vi "Auto_calibrate.vi"(3 "Mode":T4, 5 "Traverse line":T5 {"Carrier_2 Q (l/min)" format="%#.2f"; "Row Duration (mins)" format="%#.1f"; "Row No" min=0; "Trace Gas Concentration (%)" min=0.0 format="%#_4f"; "Carrier_1 Q (l/min)" format="%#.2f"; "Tunnel Speed" format="%#.2f"; "Start X" format="%#.2f"; "Start Y" format="%#.2f"; "Start Z" format="%#.2f"; "End X" format="%#.2f"; "End Y" format="%#.2f"; "End Z" format="%#.2f"; "Averaging time (min)" min=0.0 format="%#.2f"}) -> (0 "Error Messages":string, 1 "Status":T2, 2 "Traverse Out":T5 {"Carrier_2 Q (l/min)" format="%#.2f"; "Row Duration (mins)" format="%#.1f"; "Row No" min=0; "Trace Gas Concentration (%)" min=0.0 format="%#_4f"; "Carrier_1 Q (l/min)" format="%#.2f"; "Tunnel Speed" format="%#.2f"; "Start X" format="%#.2f"; "Start Y" format="%#.2f"; "Start Z" format="%#.2f"; "End X" format="%#.2f"; "End Y" format="%#.2f"; "End Z" format="%#.2f"; "Averaging time (min)" min=0.0 format="%#.2f"})   [LabVIEW 2015]
uses:
  Gen Trav/Traverse_cluster.ctl
  Gen Trav/Spacing.ctl
  Controls/Multi_run_mode.ctl
  Controls/User_Specific_mode.ctl
  Controls/Auto_Calib_Type.ctl
  Gen Trav/Multi_Run_Status.ctl
  Controls/Auto_Calib_Case.ctl
  File/Setup_Filetype.ctl
  Calibration/Calib_mode.ctl
  ADAM Client/Sub VIs/ADAM Controls/Valco_valve_ph.ctl
  ADAM Client/Sub VIs/ADAM Controls/Client_Source_Status.ctl
  Controls/Setup.ctl
  Controls/Post_Process.ctl
  Controls/Save_Data.ctl
  Controls/App_Global.ctl
  <vilib>/Analysis/baseanly.llb/Mean (DBL).vi
  Globals/Preference_global.vi
  Globals/Meas_global.vi
  Globals/Calib_global.vi
  Globals/Trav_pos_global.vi
  Globals/Gas_management_global.vi
  Globals/Extra_Commands_Global.vi
  <vilib>/Analysis/NI_AALBase.lvlib
  <vilib>/Analysis/NI_AALPro.lvlib
panel:
  out "Mix_own_Calib_Gases":bool
  out "Slope":dbl[](array[numeric])
  out "Minimum St Dev":dbl[](array[numeric])
  out "Wait factor":dbl
  out "Orig Calib file string":string
  out "Concentrations":dbl[](array[numeric])
  out "FFID St Dev":dbl[][](array[numeric]) format="%.2f"
  in  "Clear Calib History":bool
  out "Coefficients":dbl[][](array[numeric]) format="%.2f"
  out "Currently in Case":T1
  out "Valve position":dbl format="%.2f"
  out "Currently On":i32
  out "Values":dbl[][](array[numeric]) format="%.2f"
  out "FF Indexes":i16[](array[numeric])
  out "Ch No's":i16[](array[numeric])
  out "No of Calib Points":i32
  out "Root Name":string[](array[string])
  out "Calibration varying":T3
  in  "stop":bool
  out "New Calib Filenames":path[](array[path])
  # "Specific Argument Options\n      Tunnel Speed;1;2;3;4\nOR  Traverse Position\nOR   Concentration"
  # "X           Y            Z"
  # "Start"
  # "End"
  # "X           Y            Z"
  # "Start"
  # "End"
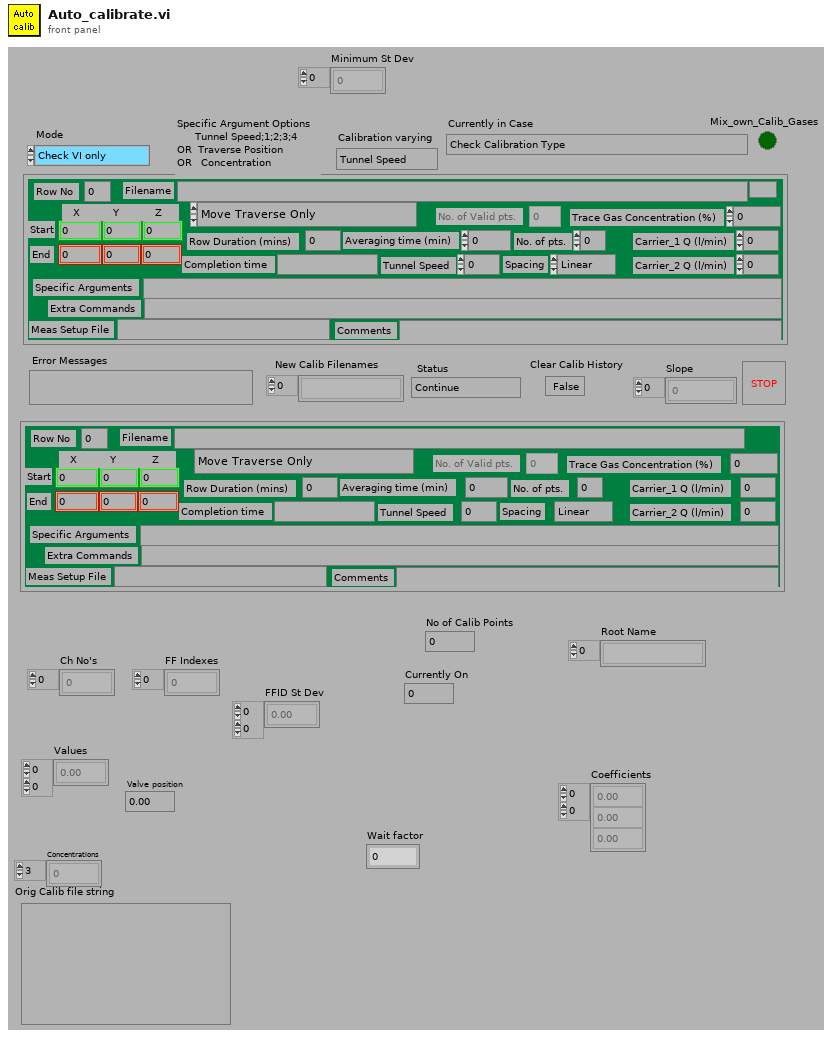
[diagram p1: front panel]
types:
  T1 = typedef "Auto_Calib_Case.ctl" = enum16{"Check Calibration Type", "Check if Original Calib file is Valid", "Get sampling rate etc. from meas setup file", "Setup Calibration Program", "Get Channel Numbers", "Check use latest selected on Mesurement setup files", "Create New Calib Filenames", "Setup Calibration Values in 2D array", "Create Measurement Setup File (Concentration Only)", "Are There Enough Calibration Points", "Set Measurement Conditions", "Measure Calibration Point", "Do Another Calibration Point?", "Skip Next Frame?", "Insert New calibration Filenames into Measurement Setup file", "Warn if FFID calibration is very non linear", "Warn if FFID variance is high", "Insert Bkgnd Variance into calib file", "Warn if FFID voltages are too low", "Warn if Current Calibration fit is poor", "Warn if Calibration Coefficients have significantly altered", "End"}
  T2 = typedef "Multi_Run_Status.ctl" = enum16{"Continue", "Jump to Next Point", "Jump to Next Row", "Jump To Fall Back", "Terminate Run"}
  T3 = typedef "Auto_Calib_Type.ctl" = enum16{"Tunnel Speed", "Traverse Position", "Concentration"}
  T4 = typedef "User_Specific_mode.ctl" = enum16{"Check VI only", "Run VI"}
  T5 = typedef "Traverse_cluster.ctl" = cluster{"Start X":sgl, "Start Y":sgl, "Start Z":sgl, "End X":sgl, "End Y":sgl, "End Z":sgl, "No. of pts.":i32, "Spacing":T6, "Filename":path, "Tunnel Speed":dbl, "Averaging time (min)":dbl, "Extra Commands":string, "Carrier_1 Q (l/min)":dbl, "Carrier_2 Q (l/min)":dbl, "Trace Gas Concentration (%)":dbl, "Specific Arguments":string, "Comments":string, "Row No":i32, "Row Type Selector":T7, "Completion time":string, "Row Duration (mins)":dbl, "No. of Valid pts.":i32, "Meas Setup File":string}
  T6 = typedef "Spacing.ctl" = enum16{"Linear", "Log", "Gauss", "Specified", "N/A"}
  T7 = typedef "Multi_run_mode.ctl" = enum16{"Move Traverse Only", "Set Tunnel Speed Only", "Set Source Only", "Set Measurement Conditions", "Single Measurement", "Vertical Profile", "Lateral Profile", "Longitudinal Profile", "Explore Volume", "Multi-Axis Profile", "Auto Calibrate", "Meas Fast FID Bkgnd", "Check Beam Power", "Scanning Valve Measurement", "Run VI Named:", "Set ADAM Ch", "Wait (minutes)", "Send Message", "Synchronize With:", "Fall Back to this Row", "Turn Off Row Repeating", "Blank Row", "Traverse 3D Volume"}
  T8 = typedef "Setup_Filetype.ctl" = enum16{"Measurement Setups", "Calibration Setups", "General", "Results File Plotter Setups", "Speed Calib Tweaks"}
  T9 = typedef "Calib_mode.ctl" = enum16{"Show Setup", "Take a New Calibration Point", "Refit Curve", "Setup Front Panel"}
  T10 = typedef "Client_Source_Status.ctl" = enum16{"Not Using", "Using", "Must Have"}
  T11 = typedef "Save_Data.ctl" = enum16{"Save No Data", "Save Data"}
  T12 = typedef "Post_Process.ctl" = enum16{"Take New Data", "Post Process Raw Data File"}
  T13 = typedef "Setup.ctl" = enum16{"Run Program", "Show Setup", "Save Current Setup", "Setup Front Panel"}
  T14 = typedef "App_Global.ctl" = enum16{"Read Global", "Write to Global", "Initialise Array"}
  T15 = typedef "Cal_Inst_type.ctl" = enum16{"Propeller anemometer", "Pressure Transducer", "Hot wire", "Cross wire velocity", "Cross wire angle", "Generic Linear", "Generic Polynomial", "Generic BackPoly", "Fast FID", "Thermocouple", "Cold wire", "Pulsed Wire"}
  T16 = typedef "Ref_Inst_type.ctl" = enum16{"Propellor anemometer", "Pressure Transducer", "Raw voltage", "Pitot-static tube", "Preston tube", "Generic Linear", "Generic Polynomial", "Thermocouple", "LDA", "Enter Value", "ADAM Channel"}
  T17 = cluster{"2nd Ref type":T16, "2nd inst present":bool}
  T18 = cluster{"high limit (10V)":sgl, "low limit (-10V)":sgl, "Ch No":i16, "Var name":string}[]
  T19 = cluster{"high limit (10V)":sgl, "low limit (-10V)":sgl, "Ch No":i16, "Var name":string}
  T20 = typedef "Inst_type.ctl" = enum16{"Propeller anemometer", "Raw voltage", "Pressure Transducer", "Pitot-static tube", "Preston tube", "Hot wire", "Cross wire 1", "Cross wire 2", "Generic Linear", "Generic Polynomial", "Generic BackPoly", "Fast FID", "Thermocouple", "Cold wire", "Pulsed Wire", "LDA Vel", "LDA Tran time", "LDA Arr time", "Microphone"}
  T21 = cluster{"high limit (10V)":sgl, "low limit (-10V)":sgl, "Ch No":i16, "Calib filename":path, "Inst type":T20, "Symbol":string, "Move channel":bool, "Use Latest":bool, "D":dbl, "Ch Name":string}[]
  T22 = typedef "Valco_valve_ph.ctl" = u16
  T23 = typedef "Status_Cluster.ctl" = cluster{"Status":T2, "Error Type":string, "Error Description":string}
  T24 = typedef "Time_Trace_Cluster.ctl" = cluster{"Weighting":dbl[], "Time (s)":dbl[], "Voltage":dbl[], "Eng Values":dbl[]}
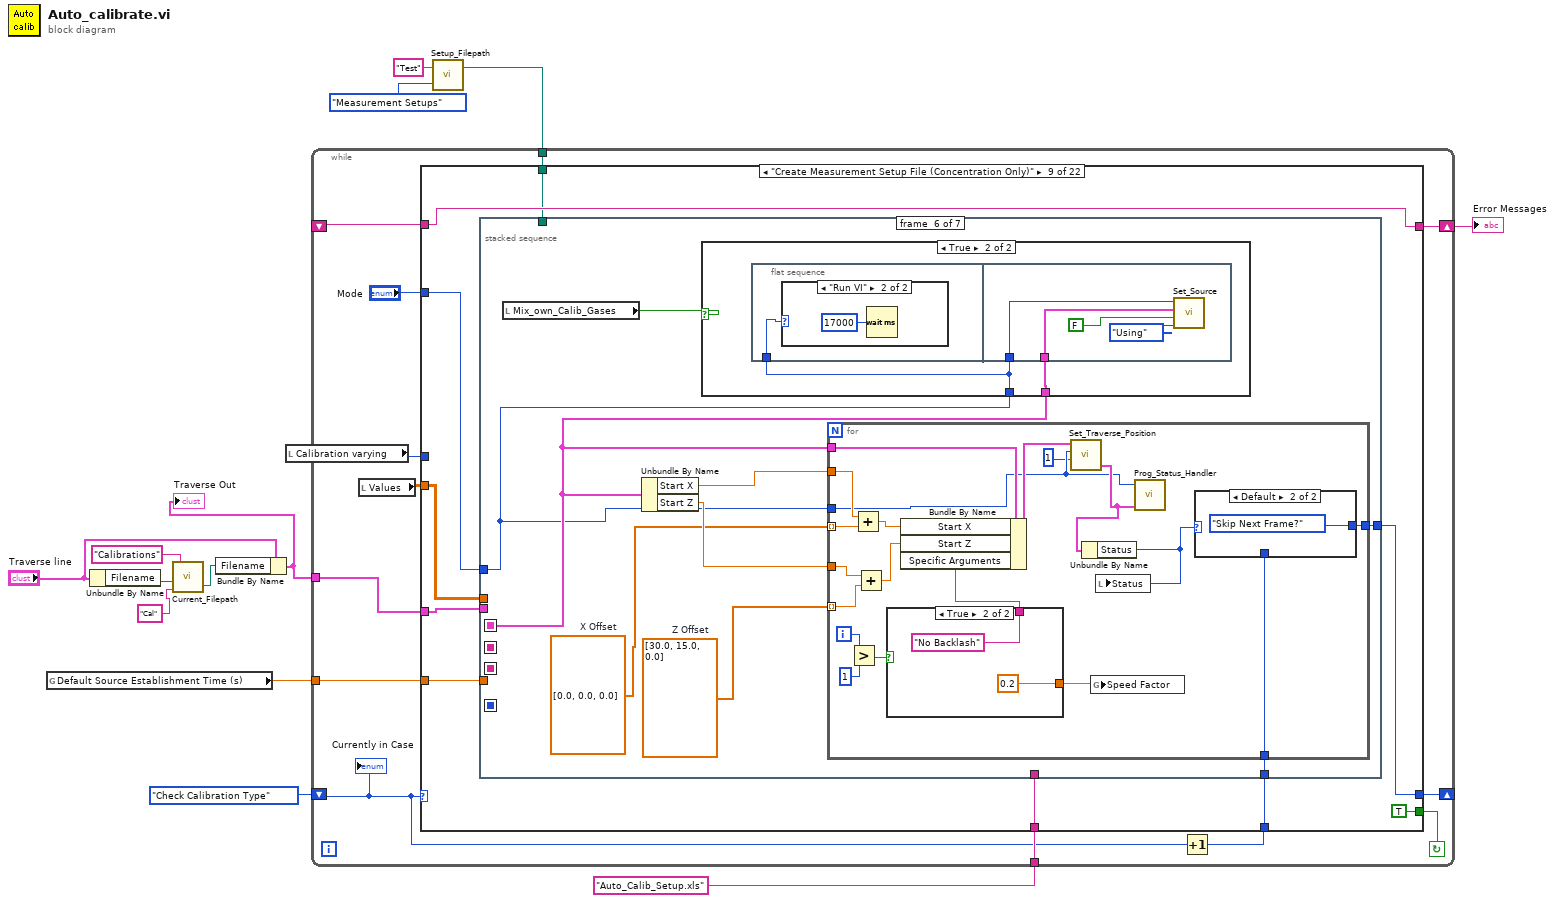
[diagram p0: block diagram]
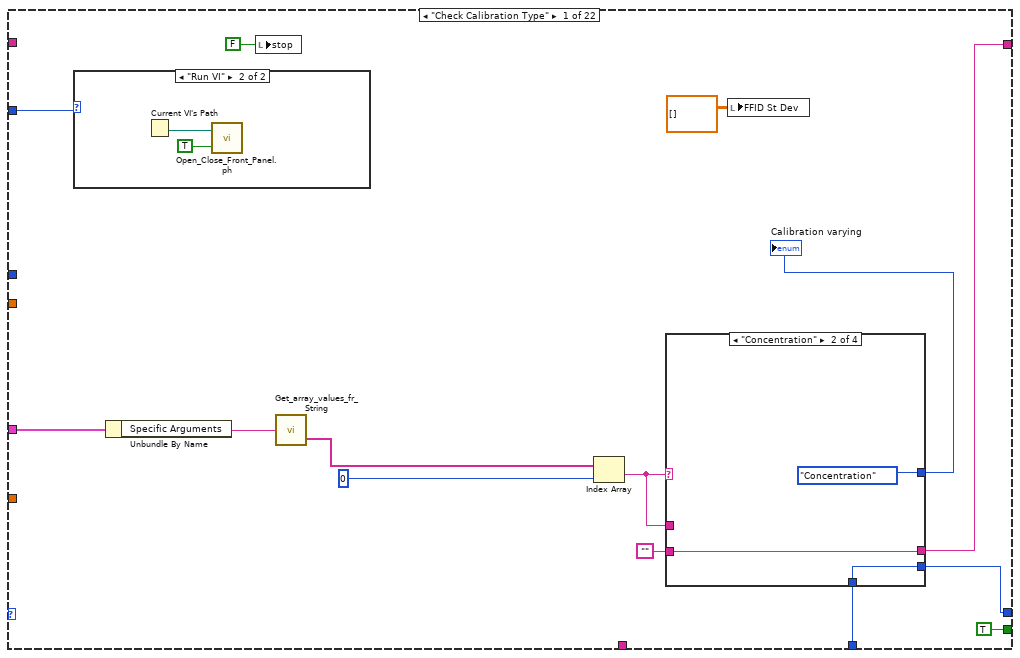
[diagram p2: hidden frame]
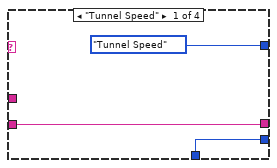
[diagram p4: hidden frame]
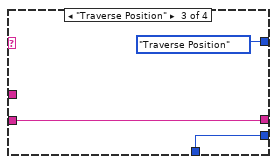
[diagram p5: hidden frame]
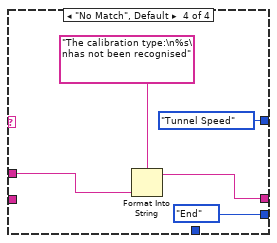
[diagram p6: hidden frame]
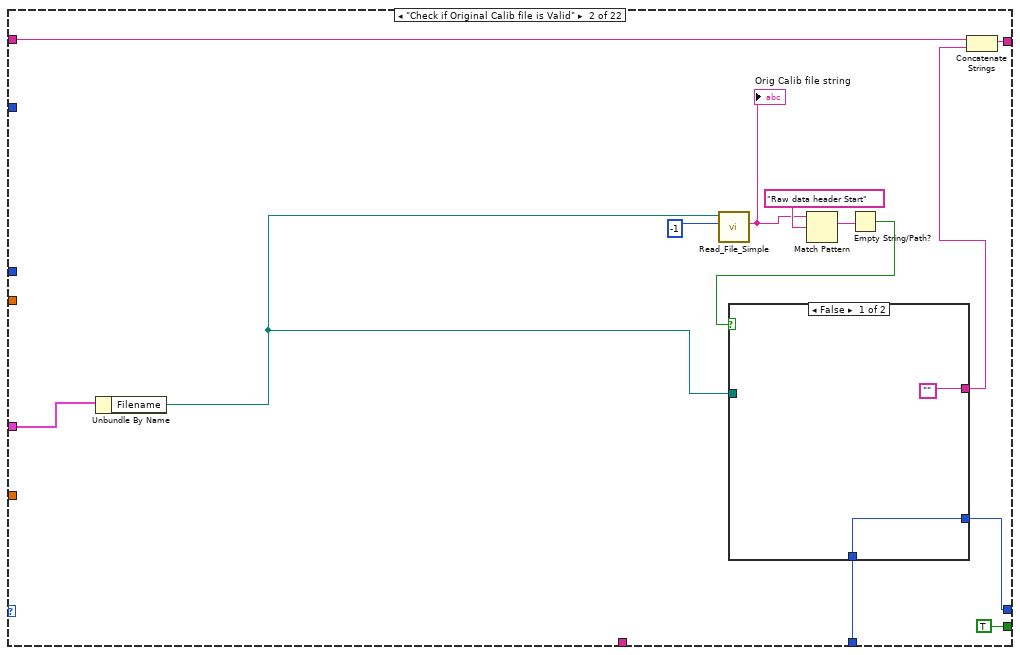
[diagram p7: hidden frame]
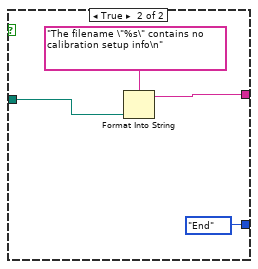
[diagram p8: hidden frame]
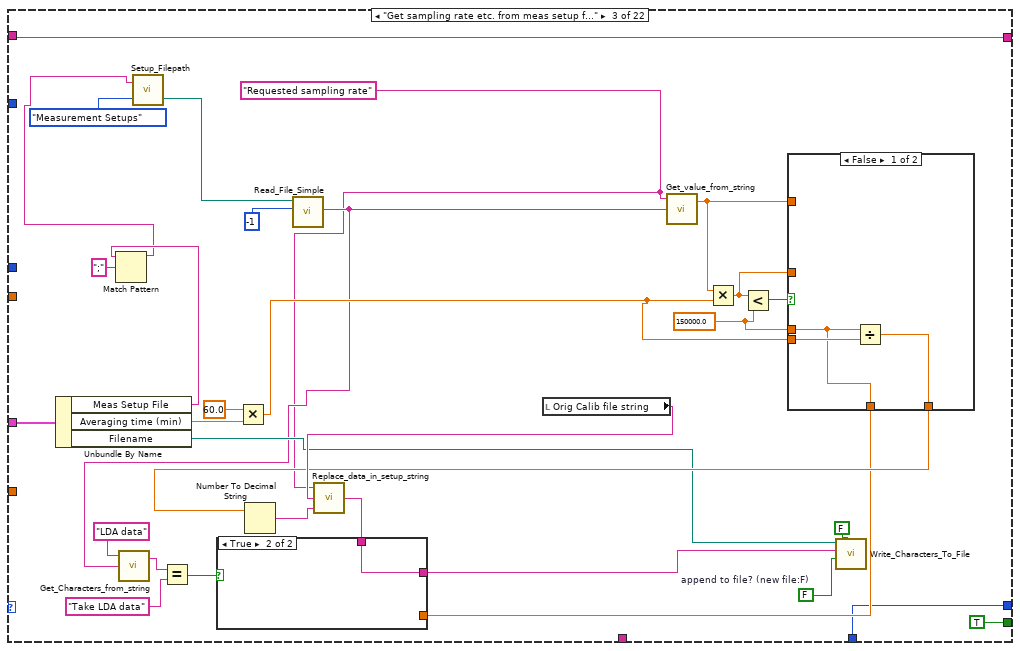
[diagram p9: hidden frame]
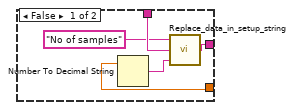
[diagram p10: hidden frame]
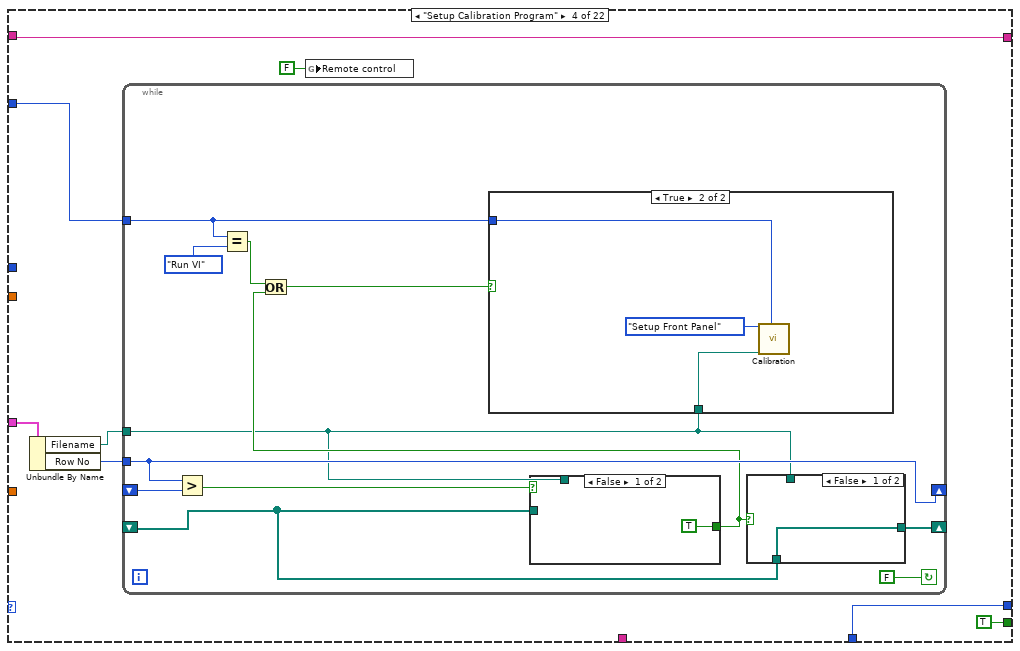
[diagram p12: hidden frame]
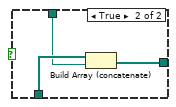
[diagram p13: hidden frame]
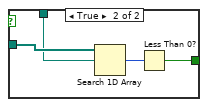
[diagram p15: hidden frame]
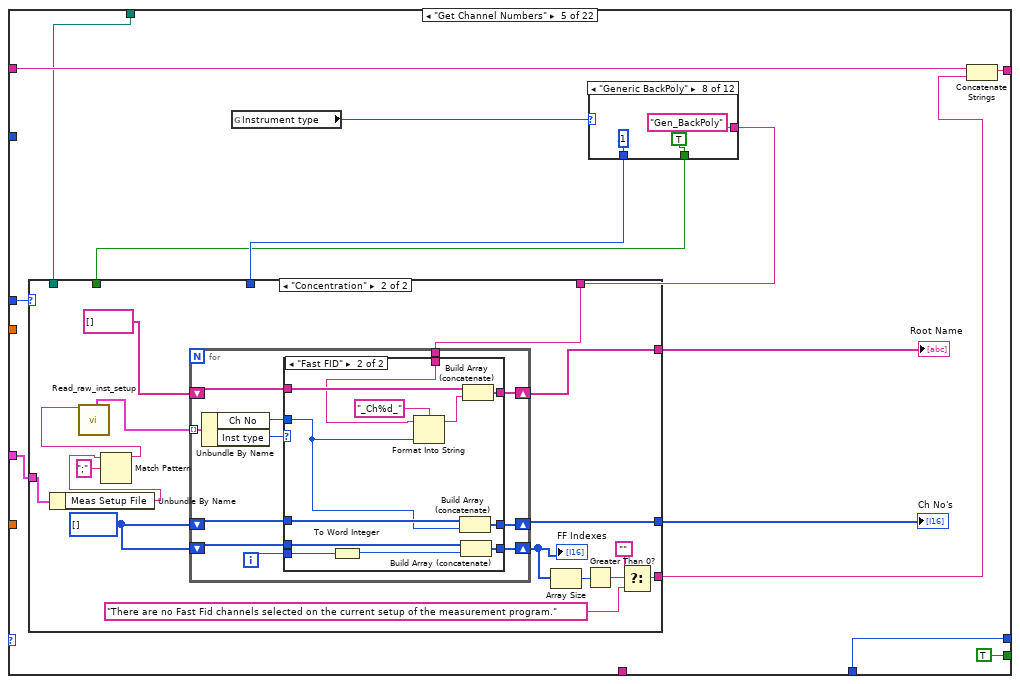
[diagram p16: hidden frame]
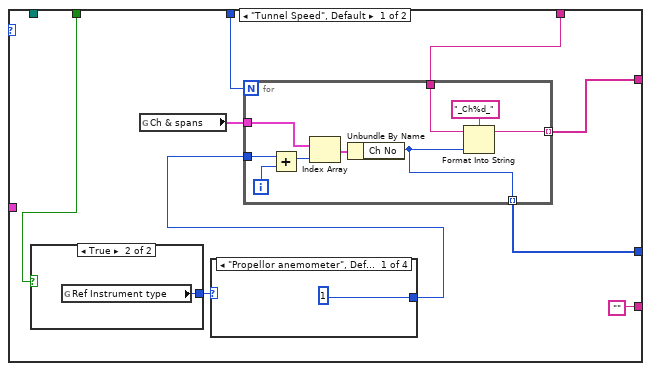
[diagram p17: hidden frame]
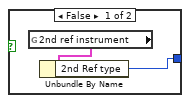
[diagram p18: hidden frame]
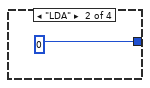
[diagram p19: hidden frame]
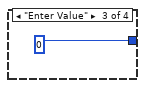
[diagram p20: hidden frame]
diagram:
  n1 = global read "Preference_global.vi" "Default Source Establishment Time (s)"() -> (w1:dbl)
  n2 = Unbundle By Name("Traverse line") -> ("Filename"=w6:path)
  n3 = call "Current_Filepath.vi"("Short_Name"="Cal" ("Data Type"), "Filename in"=w6, "Data Type"="Calibrations") -> ("Filename Out"=w5:path)  [unwired: 1 in, 1 out]
  n4 = Bundle By Name(cluster="Traverse line", "Filename"=w5) -> (w3:T5)
  "Traverse Out" <- w3
  n5 = call "Setup_Filepath.vi"("Setup File Type"=Setup_Filetype."Measurement Setups", "Filename in"="Test") -> ("Directory"=w8:path)  [unwired: 1 out]
  n6 = while {
    shift-left: _ -> [w19]
    shift-right: [w20] -> w12
    shift-left: Auto_Calib_Case."Check Calibration Type" ("Currently in Case") -> [w18]
    shift-right: [w17] -> _
    tunnel: "Auto_Calib_Setup.xls" -> [w26]
    tunnel: w8 -> [w16]
    tunnel: w3 -> [w15]
    tunnel: w1 -> [w14]
    stop <- w23 continue-if-true
    n7 = local read "Calibration varying"() -> (w22:T3)
    n8 = local read "Values"() -> (w21:dbl[][])
    n9 = Increment(x=w18) -> (x+1=w24:T1)
    n10 = case shown="\"Create Measurement Setup File (Concentration Only)\"" w18 {
      tunnel: w15 -> [w40 w69 w107 w122 w153 _ w321 w375 w448 _ w647 _ _ w892 _ _ _ _ _ _ w1131 w1162]
      tunnel: "Mode" -> [w31 _ _ w123 _ _ w327 _ w449 _ w642 _ w867 w893 _ _ _ _ _ _ _ w1163]
      tunnel: w26 -> [_ _ _ _ _ _ _ _ w452 _ _ w737 _ _ _ _ _ _ _ _ _ _]
      tunnel: [w29 w59 w89 w125 w156 w272 w325 w367 w444 w610 w635 w736 w868 w896 w917 w936 w974 w1039 w1055 w1110 w1154 w1167] -> w17
      tunnel: w24 -> [w30 w58 w89 w125 w156 w272 w325 w368 w443 w609 w631 w736 _ w895 w916 w936 w974 w1039 w1055 w1110 w1154 w1167]
      tunnel: [TRUE TRUE TRUE TRUE TRUE TRUE TRUE TRUE TRUE TRUE TRUE TRUE TRUE TRUE TRUE TRUE TRUE TRUE TRUE TRUE TRUE FALSE] -> w23
      tunnel: w22 -> [_ _ _ _ w160 _ w324 w373 _ _ w634 w738 w866 w894 w919 _ _ _ _ _ _ w1164]
      tunnel: w21 -> [_ _ _ _ _ _ _ _ w447 w619 w646 _ _ _ _ _ w981 _ _ _ _ w1161]
      tunnel: [w33 w61 w87 w126 w157 w273 w337 w370 w451 w613 w632 w734 w865 w899 w923 w945 w988 w1035 w1060 w1099 w1147 w1166] -> w20
      tunnel: w19 -> [_ w63 w87 w126 w159 w273 w337 w369 w451 w614 w632 w734 w865 w899 w923 w945 w988 w1035 w1060 w1099 w1147 w1166]
      tunnel: w16 -> [_ _ _ _ w152 w275 _ _ w450 _ _ _ _ _ _ _ _ _ _ _ _ _]
      tunnel: w14 -> [_ _ _ _ _ _ _ _ w446 _ w629 _ _ _ _ _ _ _ _ _ _ _]
      frame "Check Calibration Type" {
        n11 = case shown="\"Run VI\"" w31 {
          frame "Check VI only" {
          }
          frame "Run VI" {
            n12 = Current VI's Path() -> (path=w41:path)
            n13 = call "Open_Close_Front_Panel.ph.vi"("Front Panel Window:Open"=TRUE, "VI path"=w41) -> ()  [unwired: 2 out]
          }
        }
        n14 = Unbundle By Name(w40) -> ("Specific Arguments"=w39:string)
        n15 = local write "stop"(FALSE) -> ()
        n16 = call "Get_array_values_fr_String.vi"("String Value"=w39) -> ("String array"=w38:string[])  [unwired: 1 out]
        n17 = Index Array(array=w38, index=0 ("Index")) -> (element=w36:string)
        n18 = case shown="\"Concentration\"" w36 {
          tunnel: [Auto_Calib_Type."Tunnel Speed" ("Calibration varying") Auto_Calib_Type."Concentration" ("Calibration varying") Auto_Calib_Type."Traverse Position" ("Calibration varying") Auto_Calib_Type."Tunnel Speed" ("Calibration varying")] -> w34
          tunnel: w36 -> [_ _ _ w55]
          tunnel: [w44 w47 w50 w53] -> w33
          tunnel: "" -> [w44 w47 w50 _]
          tunnel: w30 -> [w43 w46 w49 _]
          tunnel: [w43 w46 w49 Auto_Calib_Case."End" ("Currently in Case")] -> w29
          frame "Tunnel Speed" {
          }
          frame "Concentration" {
            (unwired) ""
          }
          frame "Traverse Position" {
          }
          frame "No Match", Default {
            n19 = Format Into String(format string="The calibration type:\n%s\nhas not been recognised" ("Format String"), w55) -> (resulting string=w53:string)  [unwired: 2 in, 1 out]
          }
        }
        "Calibration varying" <- w34
        n20 = local write "FFID St Dev"(dbl[][] [] ("FFID Variance")) -> ()
      }
      frame "Check if Original Calib file is Valid" {
        n21 = Unbundle By Name(w69) -> ("Filename"=w57:path)
        n22 = call "Read_File_Simple.vi"("Filename"=w57, "number of characters (all:-1)"=-1) -> ("string"=w66:string)  [unwired: 1 in, 7 out]
        "Orig Calib file string" <- w66
        n23 = Match Pattern(string=w66, regular expression="Raw data header Start") -> (match substring=w65:string)  [unwired: 4 out]
        n24 = Empty String/Path?(string/path=w65) -> (empty?=w64:bool)
        n25 = case shown="False" w64 {
          tunnel: w57 -> [_ w75]
          tunnel: ["" w73] -> w62
          tunnel: [w70 Auto_Calib_Case."End" ("Currently in Case")] -> w59
          tunnel: w58 -> [w70 _]
          frame False {
          }
          frame True {
            n26 = Format Into String(format string="The filename \"%s\" contains no calibration setup info\n" ("Format String"), w75) -> (resulting string=w73:string)  [unwired: 2 in, 1 out]
          }
        }
        n27 = Concatenate Strings(w63, w62) -> (w61:string)
      }
      frame "Get sampling rate etc. from meas setup file" {
        w90 = FALSE  # append to file? (new file:F)
        w79 = "Requested sampling rate"
        w97 = 150000.0 ("y")
        n28 = Unbundle By Name(w107) -> ("Meas Setup File"=w85:string, "Averaging time (min)"=w105:dbl, "Filename"=w92:path)
        n29 = Match Pattern(string=w85, regular expression=";") -> (before substring=w77:string)  [unwired: 4 out]
        n30 = call "Setup_Filepath.vi"("Setup File Type"=Setup_Filetype."Measurement Setups", "Filename in"=w77) -> ("Filename Out"=w76:path)  [unwired: 1 out]
        n31 = Multiply(x=60.0, y=w105) -> (x*y=w96:dbl)
        n32 = call "Read_File_Simple.vi"("Filename"=w76, "number of characters (all:-1)"=-1) -> ("string"=w84:string)  [unwired: 1 in, 7 out]
        n33 = call "Get_Characters_from_string.vi"("Input string"=w84, "Variable name"="LDA data") -> ("Value"=w82:string)  [unwired: 1 in, 1 out]
        n34 = Equal?(x=w82, y="Take LDA data") -> (x = y?=w80:bool)
        n35 = local read "Orig Calib file string"() -> (w101:string)
        n36 = call "Get_value_from_string.vi"("Input string"=w84, "Variable name"=w79) -> ("Value"=w100:dbl)  [unwired: 1 in, 1 out]
        n37 = Multiply(x=w100, y=w96) -> (x*y=w95:dbl)
        n38 = Less?(x=w95, y=w97) -> (x < y?=w103:bool)
        n39 = case shown="False" w103 {
          tunnel: w100 -> [_ w118]
          tunnel: [w115 w118] -> w99
          tunnel: w97 -> [w114 _]
          tunnel: w96 -> [w116 _]
          tunnel: [w114 w117] -> w93
          tunnel: w95 -> [_ w117]
          frame False {
            n40 = Divide(x=w114, y=w116) -> (x/y=w115:dbl)
          }
          frame True {
          }
        }
        n41 = Number To Decimal String(number=w99) -> (decimal integer string=w98:string)  [unwired: 1 out]
        n42 = call "Replace_data_in_setup_string.vi"("New data string"=w98, "Input string"=w101, "Variable name"=w79) -> ("Appended string"=w94:string)
        n43 = case shown="True" w80 {
          tunnel: w94 -> [w112 w113]
          tunnel: w93 -> [w109 _]
          tunnel: [w108 w113] -> w91
          frame False {
            n44 = Number To Decimal String(number=w109) -> (decimal integer string=w110:string)  [unwired: 1 out]
            n45 = call "Replace_data_in_setup_string.vi"("New data string"=w110, "Input string"=w112, "Variable name"="No of samples") -> ("Appended string"=w108:string)
          }
          frame True {
          }
        }
        n46 = call "Write_Characters_To_File.vi"("file path (dialog if empty)"=w92, "advisory dialog? (display:T)"=FALSE, "character string"=w91, "append to file? (new file:F)"=w90) -> ()  [unwired: 1 in, 4 out]
      }
      frame "Setup Calibration Program" {
        n47 = Unbundle By Name(w122) -> ("Filename"=w119:path, "Row No"=w121:i32)
        n48 = while {
          shift-left: _ -> [w130]
          shift-right: [w129] -> _
          tunnel: w121 -> [w137]
          shift-left: _ -> [w138]
          shift-right: [w137] -> _
          tunnel: w123 -> [w135]
          tunnel: w119 -> [w127]
          stop <- FALSE continue-if-true
          n49 = Greater?(x=w137, y=w138) -> (0:w136:bool)
          n50 = Equal?(x=w135, y=User_Specific_mode."Run VI" ("Mode")) -> (x = y?=w133:bool)
          n51 = case shown="False" w136 {
            tunnel: w130 -> [_ w150]
            tunnel: w127 -> [_ w149]
            tunnel: [TRUE w147] -> w131
            frame False {
            }
            frame True {
              n52 = Search 1D Array(1D array=w150, element=w149) -> (index of element=w148:i32)  [unwired: 1 out]
              n53 = Less Than 0?(x=w148) -> (x < 0?=w147:bool)
            }
          }
          n54 = Or(x=w133, y=w131) -> (x .or. y?=w132:bool)
          n55 = case shown="True" w132 {
            tunnel: w135 -> [_ w145]
            tunnel: w127 -> [_ w144]
            frame False {
            }
            frame True {
              n56 = call "Calibration.vi"("Mode"=Calib_mode."Setup Front Panel", "Calib file"=w144, "Simulate/Run"=w145) -> ()  [unwired: 17 out]
            }
          }
          n57 = case shown="False" w131 {
            tunnel: w130 -> [w139 w142]
            tunnel: w127 -> [_ w141]
            tunnel: [w139 w140] -> w129
            frame False {
            }
            frame True {
              n58 = Build Array (concatenate)(w142, w141) -> (w140:path[])
            }
          }
        }
        n59 = global write "Meas_global.vi" "Remote control"(FALSE ("Remote control")) -> ()
      }
      frame "Get Channel Numbers" {
        n60 = global read "Calib_global.vi" "Instrument type"() -> (w164:T15)
        n61 = case shown="\"Generic BackPoly\"" w164 {
          tunnel: ["Prop" "Mano" "HW" "XW" "XW" "Gen_Lin" "Gen_Poly" "Gen_BackPoly" "FF" "Therm" "CW" "PWA"] -> w163
          tunnel: [1 1 1 2 2 1 1 1 1 1 1 1] -> w154
          tunnel: [TRUE TRUE TRUE TRUE FALSE TRUE TRUE TRUE TRUE TRUE TRUE TRUE] -> w151
          frame "Propeller anemometer" {
          }
          frame "Pressure Transducer" {
          }
          frame "Hot wire" {
          }
          frame "Cross wire velocity" {
          }
          frame "Cross wire angle" {
          }
          frame "Generic Linear" {
          }
          frame "Generic Polynomial" {
          }
          frame "Generic BackPoly" {
          }
          frame "Fast FID" {
          }
          frame "Thermocouple" {
          }
          frame "Cold wire" {
          }
          frame "Pulsed Wire" {
          }
        }
        n62 = case shown="\"Concentration\"" w160 {
          tunnel: w163 -> [w171 w205]
          tunnel: [w167 w204] -> w162
          tunnel: [w168 w202] -> w161
          tunnel: ["" w195] -> w158
          tunnel: w154 -> [w169 _]
          tunnel: w153 -> [_ w194]
          tunnel: w152 -> [_ _]
          tunnel: w151 -> [w165 _]
          frame "Tunnel Speed", Default {
            n63 = case shown="True" w165 {
              tunnel: [w174 w176] -> w173
              frame False {
                n64 = global read "Calib_global.vi" "2nd ref instrument"() -> (w175:T17)
                n65 = Unbundle By Name(w175) -> ("2nd Ref type"=w174:T16)
              }
              frame True {
                n66 = global read "Calib_global.vi" "Ref Instrument type"() -> (w176:T16)
              }
            }
            n67 = global read "Calib_global.vi" "Ch & spans"() -> (w170:T18)
            n68 = case shown="\"Propellor anemometer\", Default" w173 {
              tunnel: [1 i16 0 0 0] -> w166
              frame "Propellor anemometer", Default {
              }
              frame "LDA" {
              }
              frame "Enter Value" {
              }
              frame "ADAM Channel" {
              }
            }
            n69 = for {
              N: w169 -> [_]
              tunnel: [w183] -> w168 mode=indexing
              tunnel: w171 -> [w182]
              tunnel: w170 -> [w181]
              tunnel: [w180] -> w167 mode=indexing
              tunnel: w166 -> [w178]
              i -> [w179]
              n70 = Add(x=w178, y=w179) -> (x+y=w177:i32)
              n71 = Index Array(array=w181, index=w177) -> (element=w185:T19)
              n72 = Unbundle By Name(w185) -> ("Ch No"=w183:i16)
              n73 = Format Into String(format string="_Ch%d_" ("Format String"), initial string=w182, w183) -> (resulting string=w180:string)  [unwired: 1 in, 1 out]
            }
          }
          frame "Concentration" {
            w201 = i16[] []
            n74 = Unbundle By Name(w194) -> ("Meas Setup File"=w191:string)
            n75 = Match Pattern(string=w191, regular expression=";") -> (before substring=w190:string)  [unwired: 4 out]
            n76 = call "Read_raw_inst_setup.vi"("Setup file"=w190) -> ("Ch & spans choices"=w193:T21)  [unwired: 18 out]
            n77 = for {
              tunnel: w193 -> [w216] mode=indexing
              tunnel: w205 -> [w215]
              shift-right: [w211] -> w204
              shift-left: string[] [] -> [w212]
              shift-right: [w209] -> w202
              shift-left: w201 -> [w210]
              shift-right: [w208] -> w200
              shift-left: w201 -> [w207]
              i -> [w206]
              n78 = Unbundle By Name(w216) -> ("Ch No"=w214:i16, "Inst type"=w213:T20)
              n79 = case shown="\"Fast FID\"" w213 {
                tunnel: w215 -> [_ w221]
                tunnel: w214 -> [_ w223]
                tunnel: w212 -> [w219 w231]
                tunnel: [w219 w230] -> w211
                tunnel: w210 -> [w218 w229]
                tunnel: [w218 w228] -> w209
                tunnel: w207 -> [w217 w226]
                tunnel: [w217 w227] -> w208
                tunnel: w206 -> [_ w225]
                frame "Generic Linear", Default {
                }
                frame "Fast FID" {
                  n80 = To Word Integer(number=w225) -> (16bit integer=w224:i16)
                  n81 = Format Into String(format string="_Ch%d_", initial string=w221, w223) -> (resulting string=w220:string)  [unwired: 1 in, 1 out]
                  n82 = Build Array (concatenate)(w229, w223) -> (w228:i16[])
                  n83 = Build Array (concatenate)(w226, w224) -> (w227:i16[])
                  n84 = Build Array (concatenate)(w231, w220) -> (w230:string[])
                }
              }
            }
            "FF Indexes" <- w200
            n85 = Array Size(array=w200) -> (size(s)=w199:i32)
            n86 = Greater Than 0?(x=w199) -> (x > 0?=w198:bool)
            n87 = Select(t="", s=w198, f="There are no Fast Fid channels selected on the current setup of the measurement program.") -> (s? t:f=w195:string)
          }
        }
        "Root Name" <- w162
        "Ch No's" <- w161
        n88 = Concatenate Strings(w159, w158) -> (w157:string)
      }
      frame "Check use latest selected on Mesurement setup files" {
        n89 = global read "Trav_pos_global.vi" "Measurement setup files"() -> (w268:string[])
        n90 = local read "Ch No's"() -> (w274:i16[])
        n91 = Build Array (concatenate)(w268, "Current_Setup.xls") -> (w269:string[])
        n92 = for {
          tunnel: w275 -> [w278]
          tunnel: w269 -> [w277] mode=indexing
          tunnel: w274 -> [w276]
          n93 = stacked-sequence {
            seq-local: [w279 _ _] -> [_ w285 w313]
            seq-local: [_ w283 _] -> [_ _ w311]
            tunnel: w278 -> [w282 _ w310]
            tunnel: w277 -> [w281 _ w309]
            tunnel: w276 -> [_ w284 _]
            frame #0 {
              n94 = Build Path(base path=w282, name or relative path=w281) -> (appended path=w280:path)
              n95 = call "Read_File_Simple.vi"("Filename"=w280) -> ("string"=w279:string)  [unwired: 2 in, 7 out]
            }
            frame #1 {
              n96 = while {
                shift-right: [w290] -> w283
                shift-left: w285 -> [w291]
                tunnel: w284 -> [w294]
                i -> [w298]
                stop <- w287 continue-if-true
                n97 = Increment(x=w298) -> (x+1=w292:i32)
                n98 = Format Into String(format string="An ch %d Ch No", w292) -> (resulting string=w297:string)  [unwired: 2 in, 1 out]
                n99 = call "Get_value_from_string.vi"("Input string"=w291, "Variable name"=w297) -> ("Status"=w296:enum16{"Char in string", "Char not in string"}, "Value"=w295:dbl)  [unwired: 1 in]
                n100 = To Long Integer(number=w295) -> (32bit integer=w293:i32)
                n101 = Search 1D Array(1D array=w294, element=w293) -> (index of element=w289:i32)  [unwired: 1 in]
                n102 = Greater Or Equal To 0?(x=w289) -> (x >= 0?=w288:bool)
                n103 = case shown="\"Char in string\"" w296 {
                  tunnel: [TRUE FALSE] -> w287
                  frame "Char in string" {
                  }
                  frame "Char not in string" {
                  }
                }
                n104 = And(x=w288, y=w287) -> (x .and. y?=w286:bool)
                n105 = case shown="True" w286 {
                  tunnel: w292 -> [w302 _]
                  tunnel: w291 -> [w301 w306]
                  tunnel: [w300 w306] -> w290
                  frame True {
                    n106 = Format Into String(format string="An ch %d Use latest Calib", w302) -> (resulting string=w304:string)  [unwired: 2 in, 1 out]
                    n107 = call "Replace_data_in_setup_string.vi"("New data string"="TRUE" ("Replace with"), "Input string"=w301, "Variable name"=w304) -> ("Appended string"=w300:string)
                  }
                  frame False {
                  }
                }
              }
            }
            frame #2 {
              n108 = Equal?(x=w313, y=w311) -> (x = y?=w312:bool)
              n109 = case shown="True" w312 {
                tunnel: w310 -> [w316 _]
                tunnel: w311 -> [w319 _]
                tunnel: w309 -> [w315 _]
                frame False {
                  w318 = FALSE  # append to file? (new file:F)
                  n110 = Build Path(base path=w316, name or relative path=w315) -> (appended path=w314:path)
                  n111 = call "Write_Characters_To_File.vi"("file path (dialog if empty)"=w314, "advisory dialog? (display:T)"=FALSE, "character string"=w319, "append to file? (new file:F)"=w318) -> ()  [unwired: 1 in, 4 out]
                }
                frame True {
                }
              }
            }
          }
        }
      }
      frame "Create New Calib Filenames" {
        n112 = Unbundle By Name(w321) -> ("Filename"=w320:path)
        n113 = Get Date/Time String(date format (0)=enum16{"short", "long", "abbreviated"}."short") -> (date string=w331:string)  [unwired: 3 out]
        n114 = Strip Path(path=w320) -> (stripped path=w326:path)  [unwired: 1 out]
        n115 = local read "Root Name"() -> (w323:string[])
        n116 = case shown="\"Tunnel Speed\", Default" w324 {
          tunnel: w323 -> [_ w342]
          tunnel: [1 w341] -> w322
          frame "Tunnel Speed", Default {
          }
          frame "Concentration" {
            n117 = Array Size(array=w342) -> (size(s)=w341:i32)
          }
        }
        n118 = call "Replace_Character.vi"("Replace with"="-", "Input String"=w331, "Search For"="/") -> ("Output string"=w328:string)  [unwired: 1 out]
        n119 = List Folder(path=w326) -> (filenames=w339:string[])  [unwired: 1 in, 5 out]
        n120 = To Upper Case(1:w339) -> (0:w338:string[])
        n121 = for {
          N: w322 -> [_]
          tunnel: w323 -> [w345] mode=indexing
          tunnel: w338 -> [w349]
          tunnel: w326 -> [w348]
          tunnel: [w344] -> w335 mode=indexing
          tunnel: w328 -> [w346]
          tunnel: w327 -> [w343]
          n122 = while {
            tunnel: w345 -> [w356]
            tunnel: w346 -> [w357]
            tunnel: [w352] -> w347
            tunnel: w349 -> [w359]
            i -> [w361]
            stop <- w363 continue-if-true
            n123 = Increment(x=w361) -> (x+1=w358:i32)
            n124 = Format Into String(format string="%s_%d.xls" ("Format String"), initial string=w356, w357, w358) -> (resulting string=w353:string)  [unwired: 1 in, 1 out]
            n125 = call "Replace_Character.vi"("Replace with"="_", "Input String"=w353, "Search For"=" ") -> ("Output string"=w352:string)  [unwired: 1 out]
            n126 = To Upper Case(1:w352) -> (0:w362:string)
            n127 = Search 1D Array(1D array=w359, element=w362) -> (index of element=w364:i32)  [unwired: 1 out]
            n128 = Not Equal?(x=w364, y=-1) -> (x != y?=w363:bool)
          }
          n129 = Build Path(base path=w348, name or relative path=w347) -> (appended path=w344:path)
          n130 = case shown="\"Run VI\"" w343 {
            tunnel: w344 -> [_ w350]
            frame "Check VI only" {
            }
            frame "Run VI" {
              n131 = call "Calibration.vi"("Mode"=Calib_mode."Setup Front Panel", "Calib file"=w350) -> ()  [unwired: 1 in, 17 out]
            }
          }
        }
        "New Calib Filenames" <- w335
        n132 = Index Array(array=w335, index=0 ("Index")) -> (element=w333:path)
        n133 = global write "Meas_global.vi" "Results file"(w333) -> ()
      }
      frame "Setup Calibration Values in 2D array" {
        n134 = case shown="\"Concentration\"" w373 {
          tunnel: [w385 w395 w442] -> w372
          tunnel: w375 -> [w380 w393 w441]
          tunnel: ["" "" w440] -> w371
          tunnel: w368 -> [w379 w396 w439]
          tunnel: [w378 w396 w438] -> w367
          tunnel: [dbl[] [] w394 dbl[] []] -> w366
          frame "Tunnel Speed" {
            n135 = Unbundle By Name(w380) -> ("Specific Arguments"=w383:string)
            n136 = call "Get_array_values_fr_String.vi"("String Value"=w383) -> ("Numeric Array"=w381:dbl[])  [unwired: 1 out]
            n137 = Array Subset(array=w381, index=1 ("Array Index")) -> (w377:dbl[])  [unwired: 1 in]
            n138 = for {
              tunnel: w377 -> [w387] mode=indexing
              tunnel: [w386] -> w385 mode=indexing
              n139 = Build Array(w387) -> (w386:dbl[])
            }
            n140 = Increment(x=w379) -> (x+1=w378:T1)
          }
          frame "Concentration" {
            n141 = Unbundle By Name(w393) -> ("Specific Arguments"=w392:string)
            n142 = call "Read_FFID_Auto_Calib_Setup.vi"("Specific Argument"=w392) -> ("Trace concentration %"=w388:dbl[], "Carrier 2 Q"=w389:dbl[], "Carrier 1 Q"=w390:dbl[], "Mix_own_Calib_Gases"=w391:bool)  [unwired: 1 out]
            "Mix_own_Calib_Gases" <- w391
            n143 = case shown="True" w391 {
              tunnel: [w407 w428] -> w395
              tunnel: [w398 w415] -> w394
              tunnel: w390 -> [_ w420]
              tunnel: w389 -> [_ w418]
              tunnel: w388 -> [_ w422]
              frame False {
                w403 = 0.0 ("Input Element")
                n144 = Build Array(1.0, 2.0, 3.0) -> (w408:dbl[])
                n145 = Build Array("GMU:Calibration:Gas 1", "GMU:Calibration:Gas 2") -> (w399:string[])
                n146 = call "Get_Current_Scan_client.vi"("ADAM Ch Names"=w399) -> ("Numerical Values"=w402:dbl[])  [unwired: 3 out]
                n147 = Build Array (concatenate)(w403, w403, w402, w403) -> (w398:dbl[])
                n148 = for {
                  tunnel: w408 -> [w410] mode=indexing
                  tunnel: [w409] -> w407 mode=indexing
                  n149 = Build Array(w410) -> (w409:dbl[])
                }
              }
              frame True {
                n150 = for {
                  tunnel: w422 -> [w430] mode=indexing
                  tunnel: [w432] -> w421 mode=indexing if=w429
                  tunnel: w420 -> [w432] mode=indexing
                  tunnel: [w431] -> w419 mode=indexing if=w429
                  tunnel: w418 -> [w431] mode=indexing
                  tunnel: [w430] -> w417 mode=indexing if=w429
                  n151 = Not Equal To 0?(x=w430) -> (x != 0?=w429:bool)
                }
                n152 = Index Array(array=w421) -> (element=w425:dbl)  [unwired: 1 in]
                n153 = Index Array(array=w419) -> (element=w424:dbl)  [unwired: 1 in]
                n154 = Index Array(array=w417) -> (element=w416:dbl)  [unwired: 1 in]
                n155 = Build Array (concatenate)(w425, w421) -> (w426:dbl[])
                n156 = Build Array (concatenate)(w424, w419) -> (w423:dbl[])
                n157 = Build Array (concatenate)(w416, w417) -> (w412:dbl[])
                n158 = Replace Array Subset(array=w412, new element=0.0 ("element"), index=0) -> (w411:dbl[])
                n159 = for {
                  tunnel: w426 -> [w436] mode=indexing
                  tunnel: [w435] -> w428 mode=indexing
                  tunnel: w423 -> [w434] mode=indexing
                  tunnel: w411 -> [w433] mode=indexing
                  n160 = Build Array(w436, w434, w433) -> (w435:dbl[])
                }
                n161 = Multiply(x=10000.0, y=w411) -> (x*y=w415:dbl[])
              }
            }
          }
          frame "Traverse Position" {
            n162 = call "Create_Pos_array.vi"("Traverse line"=w441) -> ("Error Messages"=w440:string, "Array of Positions"=w442:dbl[][])  [unwired: 5 in, 2 out]
            n163 = Increment(x=w439) -> (x+1=w438:T1)
          }
        }
        "Values" <- w372
        "Concentrations" <- w366
        n164 = Concatenate Strings(w369, w371) -> (w370:string)
      }
      frame "Create Measurement Setup File (Concentration Only)" {
        n165 = stacked-sequence {
          seq-local: [_ w467 _ _ _ _ _] -> [_ _ w486 _ _ _ _]
          seq-local: [_ _ w484 _ _ _ _] -> [_ _ _ w507 _ _ _]
          seq-local: [_ _ _ _ w519 _ _] -> [_ _ _ _ _ _ _]
          seq-local: [_ _ _ _ w515 _ _] -> [_ _ _ _ _ w554 _]
          tunnel: w450 -> [_ w458 _ w508 _ _ _]
          tunnel: w452 -> [_ _ _ w509 _ _ _]
          tunnel: w449 -> [_ _ _ _ w518 w553 w594]
          tunnel: w448 -> [_ w464 _ _ w516 _ _]
          tunnel: w447 -> [_ _ _ _ w520 _ _]
          tunnel: w446 -> [_ _ _ _ _ _ _]
          tunnel: [_ _ _ _ _ w552 _] -> w444
          tunnel: w443 -> [_ _ _ _ _ w551 _]
          frame #0 {
            n166 = global read "Gas_management_global.vi" "Source Live"() -> (w453:bool)
            n167 = case shown="True" w453 {
              frame False {
              }
              frame True {
                w454 = u32 1  # Time to hold source OFF (microseconds)
                w455 = u32 0  # Time to hold source ON (microseconds)
                n168 = call "Arduino_Timed_Release.vi"("Time to hold source ON (microseconds)"=w455, "Time to hold source OFF (microseconds)"=w454, "Number of cycles"=u16 1) -> ()  [unwired: 2 out]
              }
            }
          }
          frame #1 {
            w471 = TRUE  # Show Dialog?
            n169 = Unbundle By Name(w464) -> ("Meas Setup File"=w465:string)
            n170 = Match Pattern(string=w465, regular expression=";") -> (before substring=w463:string)  [unwired: 4 out]
            n171 = Build Path(base path=w458, name or relative path=w463) -> (appended path=w472:path)
            n172 = Format Into String(format string="Meas Setup File   %s", w458) -> (resulting string=w457:string)  [unwired: 2 in, 1 out]
            n173 = call "Read_spec_No_of_Characters.vi"("Filename"=w472) -> ("character string"=w473:string)  [unwired: 1 out]
            n174 = call "Get_string_subset.vi"("String Name"=w457, "Show Dialog?"=w471, "String to split"=w473, "File Label"="Raw data header") -> ("Output string"=w460:string)  [unwired: 1 out]
            n175 = call "Get_value_from_string.vi"("Input string"=w460, "Variable name"="No of analogue inst") -> ("Value"=w461:dbl)  [unwired: 1 in, 1 out]
            n176 = for {
              N: w461 -> [_]
              shift-right: [w475] -> w470
              shift-left: w460 -> [w477]
              i -> [w481]
              n177 = Increment(x=w481) -> (x+1=w480:i32)
              n178 = Number To Decimal String(number=w480) -> (decimal integer string=w483:string)  [unwired: 1 out]
              n179 = Concatenate Strings("An ch ", w483, " Inst type") -> (w478:string)
              n180 = call "Replace_data_in_setup_string.vi"("New data string"="Raw voltage", "Input string"=w477, "Variable name"=w478) -> ("Appended string"=w475:string)
            }
            n181 = call "Replace_data_in_setup_string.vi"("New data string"="No LDA data", "Input string"=w470, "Variable name"="LDA data" ("Label for characters")) -> ("Appended string"=w467:string)
          }
          frame #2 {
            n182 = global read "Calib_global.vi" "New Setup String"() -> (w487:string)
            n183 = for {
              N: 4 -> [_]
              shift-right: [w492] -> w484
              shift-left: w486 -> [w493]
              tunnel: w487 -> [w489]
              i -> [w491]
              n184 = case shown="3" w491 {
                tunnel: [w496 w499 w502 "No of blocks"] -> w490
                tunnel: w489 -> [w495 w498 w501 _]
                tunnel: [w494 w497 w500 "1" ("Value")] -> w488
                frame 0, Default {
                  w496 = "No of samples"
                  n185 = call "Get_Characters_from_string.vi"("Input string"=w495, "Variable name"=w496) -> ("Value"=w494:string)  [unwired: 1 in, 1 out]
                }
                frame 2 {
                  w499 = "Actual sampling rate"
                  n186 = call "Get_Characters_from_string.vi"("Input string"=w498, "Variable name"=w499) -> ("Value"=w497:string)  [unwired: 1 in, 1 out]
                }
                frame 3 {
                  w502 = "Board type"
                  n187 = call "Get_Characters_from_string.vi"("Input string"=w501, "Variable name"=w502) -> ("Value"=w500:string)  [unwired: 1 in, 1 out]
                }
                frame 1 {
                }
              }
              n188 = call "Replace_data_in_setup_string.vi"("New data string"=w488, "Input string"=w493, "Variable name"=w490) -> ("Appended string"=w492:string)
            }
          }
          frame #3 {
            w513 = FALSE  # advisory dialog? (display:T)
            w514 = FALSE  # append to file? (new file:F)
            n189 = call "Remove_Plug_Ins_etc.vi"("Input String"=w507) -> ("Output string"=w506:string)
            n190 = call "Add_label_to_string.vi"("String to write"=w506, "File Label"="Raw data header") -> ("Output string"=w510:string)
            n191 = Build Path(base path=w508, name or relative path=w509) -> (appended path=w505:path)
            n192 = call "Add_length_to_string.vi"("String in"=w510) -> ("String out"=w512:string)
            n193 = call "Write_Characters_To_File.vi"("file path (dialog if empty)"=w505, "advisory dialog? (display:T)"=w513, "character string"=w512, "append to file? (new file:F)"=w514) -> ()  [unwired: 1 in, 4 out]
          }
          frame #4 {
            n194 = local read "Mix_own_Calib_Gases"() -> (w517:bool)
            n195 = case shown="\"Run VI\"" w518 {
              tunnel: w520 -> [w525 _]
              tunnel: [w524 u32 0 ("millisecond timer value")] -> w519
              tunnel: w517 -> [w523 _]
              tunnel: w516 -> [w522 w550]
              tunnel: [w521 w550] -> w515
              frame "Run VI" {
                n196 = case shown="True" w523 {
                  tunnel: w525 -> [w528 w547]
                  tunnel: [w527 w542] -> w524
                  tunnel: w522 -> [w526 w544]
                  tunnel: [w526 w543] -> w521
                  frame False {
                    n197 = flat-sequence {
                      tunnel: w528 -> [w530]
                      tunnel: [w532] -> w527
                      frame #0 {
                        w531 = 0 ("Index")
                        n198 = Index Array(array=w530, index (row)=w531, index (col)=w531) -> (element=w529:dbl)
                        n199 = call "Fast_FID_Valve_Control.vi"("Requested Position"=w529) -> ()  [unwired: 7 out]
                      }
                      frame #1 {
                        n200 = Tick Count (ms)() -> (millisecond timer value=w532:u32)
                      }
                    }
                  }
                  frame True {
                    w548 = T22 1 items=["", "Zero Air", "Calib 1", "Calib 2", "Measure"] ("Requested Position")
                    n201 = Index Array(array=w547, index (row)=0) -> (element=w545:dbl[])  [unwired: 1 in]
                    n202 = call "Fast_FID_Valve_Control.vi"("Requested Position"=w548) -> ()  [unwired: 7 out]
                    n203 = Index Array(array=w545) -> (element #1=w534:dbl, element #2=w535:dbl, element #3=w533:dbl)  [unwired: 3 in]
                    n204 = Bundle By Name(cluster=w544, "Carrier_1 Q (l/min)"=w534, "Carrier_2 Q (l/min)"=w535, "Trace Gas Concentration (%)"=w533) -> (w543:T5)
                    n205 = Tick Count (ms)() -> (millisecond timer value=w542:u32)
                    n206 = Build Array("Clean_Air:Hi-Tec:Dem Volt", "GMU:Mains Divertor:Valve") -> (w540:string[])
                    n207 = Build Array(2.0 ("element"), 1.0 ("element")) -> (w539:dbl[])
                    n208 = call "ASYNC_Adam_client.vi"("Values"=w539, "Channel Names"=w540) -> ()  [unwired: 1 in, 2 out]
                  }
                }
              }
              frame "Check VI only" {
              }
            }
          }
          frame #5 {
            w557 = dbl[] [0.0, 0.0, 0.0]  # X Offset
            w559 = dbl[] [30.0, 15.0, 0.0]  # Z Offset
            n209 = local read "Mix_own_Calib_Gases"() -> (w555:bool)
            n210 = Unbundle By Name(w554) -> ("Start X"=w556:sgl, "Start Z"=w558:sgl)
            n211 = case shown="True" w555 {
              tunnel: w554 -> [_ w561]
              tunnel: w553 -> [_ w560]
              frame False {
              }
              frame True {
                n212 = flat-sequence {
                  tunnel: w560 -> [w562]
                  tunnel: w561 -> [w567]
                  tunnel: w560 -> [w566]
                  frame #0 {
                    n213 = case shown="\"Run VI\"" w562 {
                      frame Default {
                      }
                      frame "Run VI" {
                        n214 = Wait (ms)(milliseconds to wait=u32 17000) -> ()  [unwired: 1 out]
                      }
                    }
                  }
                  frame #1 {
                    n215 = call "Set_Source.vi"("Source Status"=Client_Source_Status."Using", "Establish Exp Conditions"=FALSE, "Traverse line"=w567, "Simulate/Run"=w566) -> ()  [unwired: 6 out]
                  }
                }
              }
            }
            n216 = for {
              tunnel: w553 -> [w572]
              tunnel: w554 -> [w586]
              tunnel: w559 -> [w585] mode=indexing
              tunnel: w558 -> [w583]
              tunnel: w557 -> [w582] mode=indexing
              tunnel: w556 -> [w581]
              tunnel: [w569] -> w552
              tunnel: w551 -> [w568]
              i -> [w578]
              n217 = Greater?(x=w578, y=1) -> (0:w577:bool)
              n218 = Add(x=w581, y=w582) -> (x+y=w580:dbl)
              n219 = Add(x=w583, y=w585) -> (x+y=w584:dbl)
              n220 = case shown="True" w577 {
                tunnel: ["" "No Backlash"] -> w576
                tunnel: [1.0 ("f") 0.2 ("t")] -> w575
                frame False {
                }
                frame True {
                }
              }
              n221 = Bundle By Name(cluster=w586, "Start X"=w580, "Start Z"=w584, "Specific Arguments"=w576) -> (w574:T5)
              n222 = call "Set_Traverse_Position.vi"("Currently on Point"=1, "Simulate/Run"=w572, "Traverse line"=w574) -> ("Status Cluster"=w573:T23)  [unwired: 3 in]
              n223 = Unbundle By Name(w573) -> ("Status"=w570:T2)
              n224 = global write "Trav_pos_global.vi" "Speed Factor"(w575) -> ()
              n225 = local write "Status"(w570) -> ()
              n226 = call "Prog_Status_Handler.vi"("Status Cluster"=w573, "Simulate/Run"=w572) -> ()  [unwired: 2 out]
              n227 = case shown="Default" w570 {
                tunnel: [w587 Auto_Calib_Case."Skip Next Frame?" ("Currently in Case")] -> w569
                tunnel: w568 -> [w587 _]
                frame "Continue" {
                }
                frame Default {
                }
              }
            }
          }
          frame #6 {
            n228 = global write "Trav_pos_global.vi" "Speed Factor"(1.0 ("Speed Factor")) -> ()
            n229 = case shown="\"Run VI\"" w594 {
              frame "Check VI only", Default {
              }
              frame "Run VI" {
                n230 = while {
                  shift-right: [w606] -> _
                  shift-left: _ -> [w607]
                  tunnel: [w605] -> w600
                  stop <- TRUE stop-if-true
                  n231 = Get Date/Time In Seconds() -> (seconds since 1Jan1904=w606:timestamp)
                  n232 = Subtract(x=w606, y=w607) -> (x-y=w605:dbl)
                }
                n233 = Divide(x=w600, y=3600.0) -> (x/y=w599:dbl)
                n234 = Multiply(x=w599, y=0.2) -> (x*y=w597:dbl)
                n235 = Add(x=w597, y=0.8) -> (x+y=w595:dbl)
                n236 = In Range and Coerce(upper limit=2.0, x=w595, lower limit=1.0) -> (coerced(x)=→"Wait factor":dbl)  [unwired: 1 out]
              }
            }
          }
        }
      }
      frame "Are There Enough Calibration Points" {
        n237 = Array Size(array=w619) -> (size(s)=w620:i32[])
        n238 = Index Array(array=w620, index=0 ("Index")) -> (element=w615:i32)
        "No of Calib Points" <- w615
        n239 = Greater?(x=w615, y=1) -> (0:w616:bool)
        n240 = case shown="False" w616 {
          tunnel: ["Less than two calibration points have been specified\n" ""] -> w612
          tunnel: [Auto_Calib_Case."End" ("Currently in Case") w624] -> w610
          tunnel: w609 -> [_ w624]
          frame False {
          }
          frame True {
          }
        }
        n241 = Concatenate Strings(w614, w612) -> (w613:string)
        "Currently On" <- 1 ("Currently On")
      }
      frame "Set Measurement Conditions" {
        n242 = local read "Currently On"() -> (w630:i32)
        n243 = Decrement(x=w630) -> (x-1=w645:i32)
        n244 = Index Array(array=w646, index (row)=w645) -> (element=w644:dbl[])  [unwired: 1 in]
        n245 = case shown="\"Concentration\"" w634 {
          tunnel: w644 -> [w669 w686 w698]
          tunnel: w642 -> [_ _ w695]
          tunnel: w647 -> [w667 w682 w701]
          tunnel: [w668 w681 w693] -> w628
          tunnel: w630 -> [w664 _ w692]
          tunnel: w629 -> [_ _ w691]
          tunnel: [0.0 ("f") 5.0 ("f") w690] -> w626
          frame "Tunnel Speed" {
            n246 = Index Array(array=w669, index=0 ("Index")) -> (element=w657:dbl)
            n247 = while {
              shift-right: [w677] -> w659
              shift-left: _ -> [w676]
              tunnel: w657 -> [w679]
              tunnel: [w677] -> w666
              tunnel: [w676] -> w665
              stop <- FALSE continue-if-true
              n248 = Greater Than 0?(x=w679) -> (x > 0?=w677:bool)
            }
            n249 = Exclusive Or(1:w665, 2:w666) -> (0:w662:bool)
            n250 = Greater?(x=w664, y=1) -> (0:w661:bool)
            n251 = And(x=w662, y=w661) -> (x .and. y?=w660:bool)
            n252 = case shown="False" w659 {
              tunnel: [w671 w673] -> w658
              tunnel: w657 -> [w672 w673]
              frame False {
                n253 = Negate(x=w672) -> (-x=w671:dbl)
              }
              frame True {
              }
            }
            n254 = case shown="False" w660 {
              frame False {
              }
              frame True {
                n255 = call "Wait_Seconds_with_display.vi"("Message"="Please rotate the probe you are calibrating", "Seconds to wait"=10000.0) -> ()  [unwired: 2 out]
              }
            }
            n256 = Bundle By Name(cluster=w667, "Tunnel Speed"=w658) -> (w668:T5)
          }
          frame "Traverse Position" {
            n257 = Index Array(array=w686, index=0 ("Index")) -> (element=w685:dbl)
            n258 = Index Array(array=w686, index=1 ("Index")) -> (element=w684:dbl)
            n259 = Index Array(array=w686, index=2 ("Index")) -> (element=w683:dbl)
            n260 = Bundle By Name(cluster=w682, "Start X"=w685, "Start Y"=w684, "Start Z"=w683) -> (w681:T5)
          }
          frame "Concentration" {
            w700 = nan ("Start X")
            n261 = local read "Mix_own_Calib_Gases"() -> (w699:bool)
            n262 = Bundle By Name(cluster=w701, "Start X"=w700, "Start Y"=w700, "Start Z"=w700) -> (w694:T5)
            n263 = case shown="True" w699 {
              tunnel: w698 -> [w711 w728]
              tunnel: [w710 w716] -> w697
              tunnel: w694 -> [w709 w726]
              tunnel: [w709 w727] -> w693
              tunnel: [w706 w720] -> w690
              tunnel: w692 -> [w705 w715]
              tunnel: w691 -> [_ w724]
              frame False {
                n264 = Index Array(array=w711) -> (element=w710:dbl)  [unwired: 1 in]
                n265 = case shown="1" w705 {
                  tunnel: [0.0 20.0 20.0] -> w707
                  frame 1 {
                  }
                  frame 2, Default {
                  }
                  frame 3 {
                  }
                }
                n266 = local read "Wait factor"() -> (w708:dbl)
                n267 = Multiply(x=w708, y=w707) -> (x*y=w706:dbl)
              }
              frame True {
                n268 = Index Array(array=w728) -> (element #1=w717:dbl, element #2=w718:dbl, element #3=w719:dbl)  [unwired: 3 in]
                n269 = case shown="1" w715 {
                  tunnel: [w729 w730] -> w716
                  frame Default {
                    w729 = T22 4 items=["", "Zero Air", "Calib 1", "Calib 2", "Measure"] ("Requested Position")
                  }
                  frame 1 {
                    w730 = T22 1 items=["", "Zero Air", "Calib 1", "Calib 2", "Measure"] ("Requested Position")
                  }
                }
                n270 = Subtract(x=30.0, y=w724) -> (x-y=w722:dbl)
                n271 = Bundle By Name(cluster=w726, "Carrier_1 Q (l/min)"=w717, "Carrier_2 Q (l/min)"=w718, "Trace Gas Concentration (%)"=w719) -> (w727:T5)
                n272 = Greater Than 0?(x=w722) -> (x > 0?=w723:bool)
                n273 = Select(t=w722, s=w723, f=0.0) -> (s? t:f=w720:dbl)
              }
            }
            n274 = case shown="\"Run VI\"" w695 {
              tunnel: w697 -> [w702 w704]
              tunnel: [w702 w703] -> w696
              frame "Check VI only" {
              }
              frame "Run VI" {
                n275 = call "Fast_FID_Valve_Control.vi"("Requested Position"=w704) -> ("Achieved Posn."=w703:T22)  [unwired: 6 out]
              }
            }
            "Valve position" <- w696
          }
        }
        n276 = stacked-sequence {
          tunnel: w642 -> [w650 w652]
          tunnel: w628 -> [w649 _]
          tunnel: [w648 _] -> w627
          tunnel: w626 -> [_ w653]
          frame #0 {
            n277 = call "Set_Measurement_Conditions.vi"("Simulate/Run"=w650, "Currently on Point"=1, "Traverse line"=w649) -> ("Status Cluster"=w648:T23)  [unwired: 2 out]
          }
          frame #1 {
            n278 = case shown="\"Run VI\"" w652 {
              tunnel: w653 -> [_ w655]
              frame "Check VI only" {
              }
              frame "Run VI" {
                n279 = call "Wait_Seconds_with_display.vi"("Message"="Establishing Calibration Conditions", "Seconds to wait"=w655) -> ()  [unwired: 1 in, 1 out]
              }
            }
          }
        }
        n280 = Unbundle By Name(w627) -> ("Status"=w633:T2)
        "Status" <- w633
        n281 = Equal?(x=w633, y=Multi_Run_Status."Continue" ("Status")) -> (x = y?=w638:bool)
        n282 = Equal?(x=User_Specific_mode."Run VI" ("Mode"), y=w642) -> (x = y?=w639:bool)
        n283 = Increment(x=w631) -> (x+1=w636:T1)
        n284 = And(x=w638, y=w639) -> (x .and. y?=w637:bool)
        n285 = Select(t=w631, s=w637, f=w636) -> (s? t:f=w635:T1)
      }
      frame "Measure Calibration Point" {
        n286 = local read "Mix_own_Calib_Gases"() -> (w731:bool)
        n287 = case shown="\"Concentration\"" w738 {
          tunnel: w737 -> [_ w748]
          tunnel: [w741 w747] -> w733
          tunnel: [w739 w746] -> w732
          tunnel: w731 -> [_ w745]
          frame "Tunnel Speed", Default {
            n288 = local read "New Calib Filenames"() -> (w742:path[])
            n289 = Index Array(array=w742, index=0 ("Index")) -> (element=w743:path)
            n290 = call "Calibration.vi"("Mode"=Calib_mode."Take a New Calibration Point", "Calib file"=w743) -> ("Coefficients"=w739:dbl[][], "Status Out"=w741:T2)  [unwired: 1 in, 15 out]
          }
          frame "Concentration" {
            # "St Dev"
            # "Mean"
            n291 = stacked-sequence {
              seq-local: [_ w754 _] -> [_ _ w821]
              seq-local: [_ w753 _] -> [_ _ w820]
              seq-local: [_ w751 _] -> [_ _ w818]
              tunnel: w748 -> [_ w757 _]
              tunnel: [_ w755 _] -> w747
              tunnel: [_ _ w822] -> w746
              tunnel: w745 -> [_ w752 w819]
              frame #0 {
                n292 = global write "Meas_global.vi" "Remote control"(TRUE ("Remote control")) -> ()
                n293 = global write "Meas_global.vi" "Raw data option"(enum16{"Save raw data", "Raw data not saved"}."Save raw data" ("Raw data option")) -> ()
              }
              frame #1 {
                n294 = local read "New Calib Filenames"() -> (w758:path[])
                n295 = Index Array(array=w758, index=0 ("Index")) -> (element=w756:path)
                n296 = while {
                  tunnel: [w768] -> w755
                  tunnel: w756 -> [w767]
                  tunnel: w757 -> [w765]
                  tunnel: [w764] -> w754
                  tunnel: [w763] -> w753
                  tunnel: w752 -> [w761]
                  tunnel: [w760] -> w751
                  i -> [w762]
                  stop <- w766 continue-if-true
                  n297 = stacked-sequence {
                    seq-local: [_ w772 _ _] -> [_ _ _ w811]
                    seq-local: [_ _ w781 _] -> [_ _ _ w815]
                    seq-local: [_ _ w779 _] -> [_ _ _ w807]
                    tunnel: [_ w772 _ _] -> w768
                    tunnel: w767 -> [_ w776 _ _]
                    tunnel: [_ _ _ w808] -> w766
                    tunnel: w765 -> [_ w773 _ _]
                    tunnel: [_ _ w782 _] -> w764
                    tunnel: [_ _ w781 _] -> w763
                    tunnel: w762 -> [_ _ _ w813]
                    tunnel: w761 -> [_ _ _ w799]
                    tunnel: [_ w770 _ _] -> w760
                    frame #0 {
                      n298 = global write "Meas_global.vi" "Remote control"(TRUE ("Remote control")) -> ()
                    }
                    frame #1 {
                      n299 = call "Get_Data_Base_file_code.vi"("Data Type"="Raw_Calibrations", "Results Filename"=w776, "Short_Name"="Raw_Cal" ("Data Type")) -> ("Raw Data File Name"=w770:path)  [unwired: 1 in, 3 out]
                      n300 = call "Measurement.vi"("setup"=Setup."Run Program", "Post Process"=Post_Process."Take New Data", "File"=Save_Data."Save No Data", "Raw data file"=w770, "Setup filename"=w773) -> ("Status Out"=w772:T2)  [unwired: 2 in, 12 out]
                    }
                    frame #2 {
                      n301 = local read "FF Indexes"() -> (w783:i16[])
                      n302 = global read "Meas_global.vi" "Time Trace"() -> (w780:T24[])
                      n303 = for {
                        tunnel: w783 -> [w796] mode=indexing
                        tunnel: [w795] -> w782 mode=indexing
                        tunnel: [w794] -> w781 mode=indexing
                        tunnel: w780 -> [w792]
                        tunnel: [w785] -> w779 mode=indexing
                        n304 = Index Array(array=w792, index=w796) -> (element=w791:T24)
                        n305 = Unbundle By Name(w791) -> ("Eng Values"=w784:dbl[], "Time (s)"=w790:dbl[])
                        n306 = call-poly <vilib>:"Mean.vi"("X"=w784) -> ("mean"=w788:dbl)  [unwired: 1 out]
                        n307 = Max & Min(x=w788, y=0.3) -> (max(x,y)=w786:dbl)  [unwired: 1 out]
                        n308 = Divide(x=w784, y=w786) -> (x/y=w789:dbl[])
                        n309 = call <vilib>:"Linear Fit.vi"("Y"=w789, "X"=w790) -> ("slope"=w785:dbl)  [unwired: 9 in, 4 out]
                        n310 = call "De-spiked_Stats.vi"("Raw Signal"=w784, "No of st dev to chop at"=6.0) -> ("mean"=w795:dbl, "standard deviation"=w794:dbl)  [unwired: 1 out]
                      }
                    }
                    frame #3 {
                      n311 = Select(t=0.0002, s=w799, f=6e-05) -> (s? t:f=w797:dbl)
                      n312 = Absolute Value(x=w807) -> (abs(x)=w804:dbl[])
                      n313 = Greater?(x=w804, y=w797) -> (0:w805:bool[])
                      n314 = Greater?(x=w815, y=0.15) -> (0:w814:bool[])
                      n315 = Or Array Elements(Boolean array=w805) -> (logical OR=w802:bool)
                      n316 = Or Array Elements(Boolean array=w814) -> (logical OR=w801:bool)
                      n317 = Less?(x=w813, y=4) -> (x < y?=w809:bool)
                      n318 = Equal?(x=w811, y=Multi_Run_Status."Continue" ("Status Out")) -> (x = y?=w806:bool)
                      n319 = Or(x=w802, y=w801) -> (x .or. y?=w803:bool)
                      n320 = Compound Arithmetic op=AND(w806, w803, w809) -> (w808:bool)
                      "Slope" <- w807
                    }
                  }
                }
              }
              frame #2 {
                n321 = case shown="False" w819 {
                  tunnel: [w831 w841] -> w827
                  tunnel: w818 -> [_ w845]
                  tunnel: [nan w833] -> w817
                  frame False {
                    n322 = local read "Valve position"() -> (w832:dbl)
                    n323 = local read "Concentrations"() -> (w830:dbl[])
                    n324 = Index Array(array=w830, index=w832) -> (element=w831:dbl)
                  }
                  frame True {
                    n325 = call "Read_RD_Ch_header.vi"("Raw data file"=w845) -> ("Ch Name Out"=w834:string[], "Ch Values"=w835:string[])  [unwired: 2 out]
                    n326 = Search 1D Array(1D array=w834, element="GMU:Source:Meas Strength") -> (index of element=w843:i32)  [unwired: 1 in]
                    n327 = Search 1D Array(1D array=w834, element="GMU:Source:ppm/%Density") -> (index of element=w837:i32)  [unwired: 1 in]
                    n328 = Index Array(array=w835, index=w843) -> (element=w842:string)
                    n329 = Index Array(array=w835, index=w837) -> (element=w838:string)
                    n330 = Fract/Exp String To Number(string=w842) -> (number=w840:dbl)  [unwired: 3 in, 1 out]
                    n331 = Fract/Exp String To Number(string=w838) -> (number=w833:dbl)  [unwired: 3 in, 1 out]
                    n332 = Multiply(x=10000.0, y=w840) -> (x*y=w841:dbl)
                  }
                }
                n333 = local read "FFID St Dev"() -> (w824:dbl[][])
                n334 = Build Array (concatenate)(w821, w820) -> (w823:dbl[])
                n335 = Build Array (concatenate)(w824, w823) -> (→"FFID St Dev":dbl[][])
                n336 = global read "Meas_global.vi" "Temp"() -> (w828:dbl)
                n337 = local read "New Calib Filenames"() -> (w826:path[])
                n338 = for {
                  tunnel: w821 -> [w852] mode=indexing
                  tunnel: w828 -> [w851]
                  tunnel: w827 -> [w850]
                  tunnel: [w849] -> w822 mode=indexing
                  tunnel: w826 -> [w848] mode=indexing
                  tunnel: w820 -> [w847] mode=indexing
                  tunnel: w817 -> [w846]
                  n339 = stacked-sequence {
                    tunnel: w852 -> [w858 _]
                    tunnel: w851 -> [w855 _]
                    tunnel: w850 -> [w857 _]
                    tunnel: [_ w860] -> w849
                    tunnel: w848 -> [_ w859]
                    tunnel: w847 -> [w854 _]
                    tunnel: w846 -> [w853 _]
                    frame #0 {
                      n340 = Build Array(w857, w858, w854, w853, w855) -> (w856:dbl[])
                      n341 = global write "Calib_global.vi" "Calibration Points"(w856) -> ()
                    }
                    frame #1 {
                      n342 = call "Calibration.vi"("Mode"=Calib_mode."Refit Curve", "Calib file"=w859) -> ("Coefficients"=w861:dbl[][])  [unwired: 1 in, 16 out]
                      n343 = Index Array(array=w861, index (row)=0 ("Index")) -> (element=w860:dbl[])  [unwired: 1 in]
                    }
                  }
                }
              }
            }
          }
        }
        "Coefficients" <- w732
        n344 = local write "Status"(w733) -> ()
      }
      frame "Do Another Calibration Point?" {
        n345 = local read "No of Calib Points"() -> (w877:i32)
        n346 = local read "Status"() -> (w873:T2)
        n347 = local read "Currently On"() -> (w869:i32)
        n348 = case shown="\"Terminate Run\"" w873 {
          tunnel: [w887 w888 TRUE w891] -> w875
          tunnel: [w887 w888 FALSE w891] -> w876
          frame "Continue", Default {
            w887 = TRUE
          }
          frame "Jump to Next Point" {
            w888 = TRUE
          }
          frame "Jump to Next Row" {
          }
          frame "Terminate Run" {
            w891 = FALSE
          }
        }
        n349 = Greater?(x=w877, y=w869) -> (0:w874:bool)
        n350 = Compound Arithmetic op=AND(invert "stop", w875) -> (w872:bool)
        n351 = Compound Arithmetic op=AND(w872, w876, w874) -> (w870:bool)
        n352 = case shown="False" w870 {
          tunnel: w869 -> [_ w886]
          tunnel: [w880 Auto_Calib_Case."Set Measurement Conditions" ("Currently in Case")] -> w868
          tunnel: w867 -> [w881 _]
          tunnel: w866 -> [w879 _]
          frame False {
            n353 = case shown="\"Run VI\"" w881 {
              tunnel: [Auto_Calib_Case."End" ("Currently in Case") Auto_Calib_Case."Skip Next Frame?" ("Currently in Case")] -> w880
              tunnel: w879 -> [_ _]
              frame "Check VI only" {
              }
              frame "Run VI" {
              }
            }
          }
          frame True {
            n354 = Increment(x=w886) -> (x+1=w885:i32)
            n355 = local write "Currently On"(w885) -> ()
          }
        }
        n356 = case shown="True" "stop" {
          frame False {
          }
          frame True {
            n357 = local write "Status"(Multi_Run_Status."Terminate Run" ("Status")) -> ()
          }
        }
      }
      frame "Skip Next Frame?" {
        n358 = local read "Status"() -> (w897:T2)
        n359 = case shown="\"Concentration\"" w894 {
          tunnel: w893 -> [_ w900]
          tunnel: w892 -> [_ w901]
          frame "Tunnel Speed", Default {
          }
          frame "Concentration" {
            w903 = T22 1 items=["", "Zero Air", "Calib 1", "Calib 2", "Measure"] ("Requested Position")
            n360 = local read "Mix_own_Calib_Gases"() -> (w902:bool)
            n361 = case shown="True" w902 {
              tunnel: w901 -> [_ w906]
              tunnel: w900 -> [_ w907]
              frame False {
              }
              frame True {
                w904 = 0.0 ("Carrier_1 Q (l/min)")
                n362 = Bundle By Name(cluster=w906, "Carrier_1 Q (l/min)"=w904, "Carrier_2 Q (l/min)"=w904, "Trace Gas Concentration (%)"=w904) -> (w905:T5)
                n363 = call "Set_Source.vi"("Source Status"=Client_Source_Status."Not Using", "Establish Exp Conditions"=FALSE, "Traverse line"=w905, "Simulate/Run"=w907) -> ()  [unwired: 6 out]
              }
            }
            n364 = call "Fast_FID_Valve_Control.vi"("Requested Position"=w903) -> ()  [unwired: 7 out]
          }
        }
        n365 = case shown="\"Terminate Run\", Default" w897 {
          tunnel: [w910 Auto_Calib_Case."End" ("Currently in Case")] -> w896
          tunnel: w895 -> [w910 _]
          frame "Continue" {
          }
          frame "Terminate Run", Default {
          }
        }
      }
      frame "Insert New calibration Filenames into Measurement Setup file" {
        n366 = local read "New Calib Filenames"() -> (w912:path[])
        n367 = global read "Meas_global.vi" "Raw data file"() -> (w922:path)
        n368 = local read "Ch No's"() -> (w913:i16[])
        n369 = Strip Path(path=w922) -> (stripped path=w921:path)  [unwired: 1 out]
        n370 = Equal?(x=Auto_Calib_Type."Concentration" ("Calibration varying"), y=w919) -> (x = y?=w918:bool)
        n371 = call "Current_Calib_Filenames.vi"("Calib Filename"=w912, "Channel Numbers"=w913, "Mode"=App_Global."Write to Global") -> ()  [unwired: 3 out]
        n372 = case shown="False" w918 {
          tunnel: [Auto_Calib_Case."Warn if Current Calibration fit is poor" ("Currently in Case") w929] -> w917
          tunnel: w916 -> [_ w929]
          tunnel: w912 -> [_ w928]
          tunnel: [1 w927] -> w915
          frame False {
          }
          frame True {
            n373 = Array Size(array=w928) -> (size(s)=w927:i32)
          }
        }
        n374 = for {
          N: w915 -> [_]
          tunnel: w912 -> [w931] mode=indexing
          tunnel: w921 -> [w935]
          w933 = FALSE  # Variable Target?
          n375 = Strip Path(path=w931) -> (name=w934:string)  [unwired: 1 out]
          n376 = Build Path(base path=w935, name or relative path=w934) -> (appended path=w930:path)
          n377 = call "Remember_Calib_Filenames.vi"("Filename to Remember"=w930) -> ()  [unwired: 1 out]
          n378 = call "Copy_with_Check.vi"("Mode"=enum16{"Move", "Copy"}."Copy", "Target Path"=w930, "Variable Target?"=w933, "Source Path"=w931) -> ()  [unwired: 1 out]
        }
      }
      frame "Warn if FFID calibration is very non linear" {
        w952 = FALSE  # Dialog Box (T)
        n379 = local read "Root Name"() -> (w951:string[])
        n380 = local read "Coefficients"() -> (w954:dbl[][])
        n381 = for {
          tunnel: w954 -> [w961] mode=indexing
          shift-right: [w963] -> w949
          shift-left: "" -> [w964]
          tunnel: w951 -> [w965] mode=indexing
          tunnel: [w958] -> w944 mode=indexing
          tunnel: "If the calibration fit for %s had been linear instead of a second order polynomial, it would have yielded an average fit error of %.1f%%.\\n" ("Format String") -> [w956]
          n382 = Index Array(array=w961, index=0 ("Index")) -> (element=w959:dbl)
          n383 = Absolute Value(x=w959) -> (abs(x)=w958:dbl)
          n384 = Less?(x=w958, y=2.2) -> (x < y?=w962:bool)
          n385 = case shown="False" w962 {
            tunnel: w965 -> [w967 _]
            tunnel: w958 -> [w968 _]
            tunnel: w964 -> [w971 w972]
            tunnel: [w969 w972] -> w963
            tunnel: w956 -> [w966 _]
            frame False {
              n386 = Format Into String(format string=w966, w967, w968) -> (resulting string=w970:string)  [unwired: 2 in, 1 out]
              n387 = Concatenate Strings(w971, w970) -> (w969:string)
            }
            frame True {
            }
          }
        }
        n388 = Array Max & Min(array=w944) -> (max value=w943:dbl)  [unwired: 3 out]
        n389 = Greater?(x=w943, y=7.0) -> (0:w941:bool)
        n390 = Select(t="Very Poor FFID Linearity", s=w941, f="Poor FFID Linearity") -> (s? t:f=w938:string)
        n391 = Empty String/Path?(string/path=w949) -> (empty?=w948:bool)
        n392 = Not(x=w948) -> (.not. x?=w947:bool)
        n393 = Bundle By Name(cluster=errorcluster {"status"=FALSE, "code"=0, "source"=""} ("error in (no error)"), "source"=w949, "status"=w947) -> (w946:errorcluster)
        n394 = call "EnFlo_Error_Handler.vi"("error in (no error)"=w946, "Error Type"=w938, "Dialog Box (T)"=w952) -> ()  [unwired: 3 out]
      }
      frame "Warn if FFID variance is high" {
        w994 = FALSE  # Dialog Box (T)
        n395 = local read "New Calib Filenames"() -> (w976:path[])
        n396 = local read "FFID St Dev"() -> (w996:dbl[][])
        n397 = Index Array(array=w981, index (col)=0 ("disabled index (col)")) -> (element=w979:dbl[])  [unwired: 1 in]
        n398 = Array Size(array=w976) -> (size(s)=w975:i32)
        n399 = for {
          tunnel: w996 -> [w1013]
          shift-right: [w1015] -> w992
          shift-left: "" -> [w1016]
          tunnel: w976 -> [w1004] mode=indexing
          tunnel: "For %s the measurement at %dppm had a standard deviation of %.2f volts for an average value of  %.1f volts.\\n" ("Format String") -> [w1014]
          tunnel: w979 -> [w1007]
          tunnel: [w1006] -> w977 mode=indexing
          tunnel: w975 -> [w1002]
          tunnel: [w998] -> w973 mode=indexing
          i -> [w1001]
          n400 = Add(x=w1002, y=w1001) -> (x+y=w1000:i32)
          n401 = Strip Path(path=w1004) -> (name=w1003:string)  [unwired: 1 out]
          n402 = Index Array(array=w1013, index (col)=w1001) -> (element=w1005:dbl[])  [unwired: 1 in]
          n403 = Index Array(array=w1013, index (col)=w1000) -> (element=w999:dbl[])  [unwired: 1 in]
          n404 = Array Max & Min(array=w999) -> (min value=w998:dbl)  [unwired: 3 out]
          n405 = call-poly <vilib>:"Mean.vi"("X"=w1005) -> ("mean"=w1012:dbl)  [unwired: 1 out]
          n406 = Divide(x=w999, y=w1012) -> (x/y=w1011:dbl[])
          n407 = Array Max & Min(array=w1011) -> (max value=w1006:dbl, max index (indices)=w1008:i32)  [unwired: 2 out]
          n408 = Greater?(x=w1006, y=0.06) -> (0:w1009:bool)
          n409 = case shown="True" w1009 {
            tunnel: w1003 -> [_ w1027]
            tunnel: w1016 -> [w1017 w1033]
            tunnel: [w1017 w1031] -> w1015
            tunnel: w1014 -> [_ w1030]
            tunnel: w1008 -> [_ w1028]
            tunnel: w1007 -> [_ w1029]
            tunnel: w1006 -> [_ _]
            tunnel: w999 -> [_ w1026]
            tunnel: w1005 -> [_ w1024]
            frame False {
            }
            frame True {
              n410 = local read "Concentrations"() -> (w1022:dbl[])
              n411 = Index Array(array=w1029, index=w1028) -> (element=w1023:dbl)
              n412 = Index Array(array=w1026, index=w1028) -> (element=w1020:dbl)
              n413 = Index Array(array=w1024, index=w1028) -> (element=w1025:dbl)
              n414 = Index Array(array=w1022, index=w1023) -> (element=w1021:dbl)
              n415 = Multiply(x=w1020, y=2.5) -> (x*y=w1019:dbl)
              n416 = Format Into String(format string=w1030, w1027, w1021, w1019, w1025) -> (resulting string=w1032:string)  [unwired: 2 in, 1 out]
              n417 = Concatenate Strings(w1033, w1032) -> (w1031:string)
            }
          }
        }
        "Minimum St Dev" <- w973
        n418 = Array Max & Min(array=w977) -> (max value=w987:dbl)  [unwired: 3 out]
        n419 = Greater?(x=w987, y=0.09) -> (0:w985:bool)
        n420 = Select(t="Very unstable FFID calibration point", s=w985, f="Unstable FFID calibration point") -> (s? t:f=w982:string)
        n421 = Empty String/Path?(string/path=w992) -> (empty?=w991:bool)
        n422 = Not(x=w991) -> (.not. x?=w990:bool)
        n423 = Bundle By Name(cluster=errorcluster {"status"=FALSE, "code"=0, "source"=""} ("error in (no error)"), "source"=w992, "status"=w990) -> (w989:errorcluster)
        n424 = call "EnFlo_Error_Handler.vi"("error in (no error)"=w989, "Error Type"=w982, "Dialog Box (T)"=w994) -> ()  [unwired: 3 out]
      }
      frame "Insert Bkgnd Variance into calib file" {
        n425 = local read "New Calib Filenames"() -> (w1036:path[])
        n426 = local read "Minimum St Dev"() -> (w1037:dbl[])
        n427 = local read "Coefficients"() -> (w1034:dbl[][])
        n428 = for {
          tunnel: w1037 -> [w1042] mode=indexing
          tunnel: w1036 -> [w1048] mode=indexing
          tunnel: w1034 -> [w1045] mode=indexing
          n429 = call "Read_File_Simple.vi"("Filename"=w1048) -> ("string"=w1052:string)  [unwired: 2 in, 7 out]
          n430 = Index Array(array=w1045, index=2) -> (element=w1043:dbl)
          n431 = Multiply(x=w1042, y=w1043) -> (x*y=w1041:dbl)
          n432 = Square(x=w1041) -> (x^2=w1040:dbl)
          n433 = Number To Fractional String(number=w1040, precision (6)=i16 8) -> (F-format string=w1050:string)  [unwired: 2 out]
          n434 = call "Replace_data_in_setup_string.vi"("New data string"=w1050, "Input string"=w1052, "Variable name"="Fast FID Bkgnd Variance") -> ("Appended string"=w1047:string)
          n435 = call "Write_File_Simple.vi"("append to file? (new file:F)"=FALSE, "character string"=w1047, "file path"=w1048) -> ()  [unwired: 2 out]
        }
      }
      frame "Warn if FFID voltages are too low" {
        w1066 = FALSE  # Dialog Box (T)
        n436 = local read "Coefficients"() -> (w1058:dbl[][])
        n437 = local read "Concentrations"() -> (w1053:dbl[])
        n438 = local read "New Calib Filenames"() -> (w1057:path[])
        n439 = Array Max & Min(array=w1053) -> (max value=w1054:dbl)  [unwired: 3 out]
        n440 = for {
          shift-right: [w1078] -> w1064
          shift-left: "" -> [w1079]
          tunnel: "For %s the maximum measured calibration voltage was %.1f volts.\nCheck that the FID is running and correctly connected to the acquisition system." ("Format String") -> [w1077]
          tunnel: w1058 -> [w1075] mode=indexing
          tunnel: w1057 -> [w1071] mode=indexing
          tunnel: w1054 -> [w1070]
          n441 = Split 1D Array(array=w1075, index=1) -> (second subarray=w1074:dbl[])  [unwired: 1 out]
          n442 = call "Polybackwards.vi"("Coefficients"=w1074, "Y input"=w1070) -> ("X output"=w1069:dbl)  [unwired: 1 out]
          n443 = Less?(x=w1069, y=0.2) -> (x < y?=w1072:bool)
          n444 = case shown="True" w1072 {
            tunnel: w1079 -> [w1080 w1087]
            tunnel: [w1080 w1085] -> w1078
            tunnel: w1077 -> [_ w1084]
            tunnel: w1071 -> [_ w1083]
            tunnel: w1069 -> [_ w1081]
            frame False {
            }
            frame True {
              n445 = Strip Path(path=w1083) -> (name=w1082:string)  [unwired: 1 out]
              n446 = Format Into String(format string=w1084, w1082, w1081) -> (resulting string=w1086:string)  [unwired: 2 in, 1 out]
              n447 = Concatenate Strings(w1087, w1086) -> (w1085:string)
            }
          }
        }
        n448 = Empty String/Path?(string/path=w1064) -> (empty?=w1063:bool)
        n449 = Not(x=w1063) -> (.not. x?=w1062:bool)
        n450 = Bundle By Name(cluster=errorcluster {"status"=FALSE, "code"=0, "source"=""} ("error in (no error)"), "source"=w1064, "status"=w1062) -> (w1061:errorcluster)
        n451 = call "EnFlo_Error_Handler.vi"("error in (no error)"=w1061, "Error Type"="Low FFID calibration voltages", "Dialog Box (T)"=w1066) -> ()  [unwired: 3 out]
      }
      frame "Warn if Current Calibration fit is poor" {
        w1106 = FALSE  # Dialog Box (T)
        n452 = local read "Root Name"() -> (w1105:string[])
        n453 = local read "Coefficients"() -> (w1108:dbl[][])
        n454 = local read "Mix_own_Calib_Gases"() -> (w1090:bool)
        n455 = Select(t=1.5, s=w1090, f=1.0 ("y")) -> (s? t:f=w1088:dbl)
        n456 = for {
          tunnel: w1108 -> [w1115] mode=indexing
          shift-right: [w1117] -> w1103
          shift-left: "" -> [w1118]
          tunnel: w1105 -> [w1119] mode=indexing
          tunnel: [w1112] -> w1098 mode=indexing
          tunnel: w1088 -> [w1111]
          n457 = Index Array(array=w1115, index=0 ("Index")) -> (element=w1113:dbl)
          n458 = Absolute Value(x=w1113) -> (abs(x)=w1112:dbl)
          n459 = Less?(x=w1112, y=w1111) -> (x < y?=w1116:bool)
          n460 = case shown="True" w1116 {
            tunnel: w1119 -> [w1121 _]
            tunnel: w1112 -> [w1122 _]
            tunnel: w1118 -> [w1125 w1126]
            tunnel: [w1123 w1126] -> w1117
            frame False {
              n461 = Format Into String(format string="The calibration for %s has an average fit error of %.1f%%\\n" ("Format String"), w1121, w1122) -> (resulting string=w1124:string)  [unwired: 2 in, 1 out]
              n462 = Concatenate Strings(w1125, w1124) -> (w1123:string)
            }
            frame True {
            }
          }
        }
        n463 = Array Max & Min(array=w1098) -> (max value=w1097:dbl)  [unwired: 3 out]
        n464 = Greater?(x=w1097, y=7.0) -> (0:w1095:bool)
        n465 = Select(t="Very Poor Calibration", s=w1095, f="Poor Calibration") -> (s? t:f=w1092:string)
        n466 = Empty String/Path?(string/path=w1103) -> (empty?=w1102:bool)
        n467 = Not(x=w1102) -> (.not. x?=w1101:bool)
        n468 = Bundle By Name(cluster=errorcluster {"status"=FALSE, "code"=0, "source"=""} ("error in (no error)"), "source"=w1103, "status"=w1101) -> (w1100:errorcluster)
        n469 = call "EnFlo_Error_Handler.vi"("error in (no error)"=w1100, "Error Type"=w1092, "Dialog Box (T)"=w1106) -> ()  [unwired: 3 out]
      }
      frame "Warn if Calibration Coefficients have significantly altered" {
        w1152 = FALSE  # Dialog Box (T)
        w1139 = 8.0 ("y")
        n470 = local read "New Calib Filenames"() -> (w1144:path[])
        n471 = local read "Root Name"() -> (w1143:string[])
        n472 = global read "Calib_global.vi" "Instrument type"() -> (w1142:T15)
        n473 = Unbundle By Name(w1131) -> ("Extra Commands"=w1130:string)
        n474 = global read "Extra_Commands_Global.vi" "If Command"() -> (w1132:string)
        n475 = call "Extra_Commands.vi"("String to Search"=w1130, "Command"=w1132) -> ("String Value"=w1129:string)  [unwired: 1 in, 4 out]
        n476 = call "Calibration_Analysis.vi"("Root Name"=w1143, "New Calib Filenames"=w1144, "Instrument type"=w1142, "Clear Calib History"="Clear Calib History") -> ("Error String"=w1141:string, "Max % Error"=w1127:dbl)
        n477 = call "Get_array_values_fr_String.vi"("String Value"=w1129) -> ("Numeric Array"=w1128:dbl[], "String array"=w1134:string[])
        n478 = Greater?(x=w1127, y=w1139) -> (0:w1140:bool)
        n479 = Index Array(array=w1134, index=0 ("Index")) -> (element=w1135:string)
        n480 = case shown="\"Drift Greater Than\"" w1135 {
          tunnel: w1128 -> [w1158 _]
          tunnel: w1127 -> [w1157 _]
          frame "Drift Greater Than" {
            n481 = Index Array(array=w1158, index=1 ("Index")) -> (element=w1156:dbl)
            n482 = Greater?(x=w1157, y=w1156) -> (0:w1155:bool)
            n483 = case shown="True" w1155 {
              frame False {
              }
              frame True {
                n484 = local write "Status"(Multi_Run_Status."Jump To Fall Back" ("Status")) -> ()
              }
            }
          }
          frame "No Match", Default {
          }
        }
        n485 = Format Into String(format string="Calibration Drift Greater than %d%%", w1139) -> (resulting string=w1137:string)  [unwired: 2 in, 1 out]
        n486 = Select(t=w1137, s=w1140, f="Calibration Drift") -> (s? t:f=w1145:string)
        n487 = Empty String/Path?(string/path=w1141) -> (empty?=w1150:bool)
        n488 = Not(x=w1150) -> (.not. x?=w1149:bool)
        n489 = Bundle By Name(cluster=errorcluster {"status"=FALSE, "code"=0, "source"=""} ("error in (no error)"), "source"=w1141, "status"=w1149) -> (w1148:errorcluster)
        n490 = call "EnFlo_Error_Handler.vi"("error in (no error)"=w1148, "Error Type"=w1145, "Dialog Box (T)"=w1152) -> ()  [unwired: 3 out]
      }
      frame "End" {
        n491 = case shown="\"Concentration\"" w1164 {
          tunnel: w1162 -> [_ w1170]
          tunnel: w1163 -> [_ w1169]
          tunnel: w1161 -> [_ w1168]
          frame "Tunnel Speed", Default {
          }
          frame "Concentration" {
            n492 = stacked-sequence {
              tunnel: w1170 -> [w1184 _]
              tunnel: w1169 -> [w1176 w1191]
              tunnel: w1168 -> [w1173 _]
              frame #0 {
                n493 = Unbundle By Name(w1184) -> ("Averaging time (min)"=w1186:dbl)
                n494 = global read "Trav_pos_global.vi" "Simulation Time"() -> (w1179:timestamp)
                n495 = Unbundle By Name(w1184) -> ("Start X"=w1171:sgl, "Start Z"=w1175:sgl)
                n496 = Array Size(array=w1173) -> (size(s)=w1174:i32[])
                n497 = Index Array(array=w1174) -> (element=w1172:i32)  [unwired: 1 in]
                n498 = Multiply(x=60.0, y=w1186) -> (x*y=w1183:dbl)
                n499 = Add(x=w1175, y=50.0) -> (x+y=w1187:dbl)
                n500 = Add(x=w1183, y=60.0) -> (x+y=w1181:dbl)
                n501 = Bundle By Name(cluster=w1184, "Start X"=w1171, "Start Z"=w1187) -> (w1188:T5)
                n502 = Multiply(x=w1181, y=w1172) -> (x*y=w1180:dbl)
                n503 = Add(x=w1179, y=w1180) -> (x+y=w1177:timestamp)
                n504 = call "Set_Traverse_Position.vi"("Currently on Point"=1, "Simulate/Run"=w1176, "Traverse line"=w1188) -> ()  [unwired: 3 in, 1 out]
                n505 = call "Run_FFID_Bkgnd.vi"("Simulated Time"=w1177, "Run Now?"=TRUE, "Simulate/Run"=w1176) -> ()  [unwired: 3 out]
              }
              frame #1 {
                n506 = case shown="\"Run VI\"" w1191 {
                  frame "Check VI only", Default {
                  }
                  frame "Run VI" {
                    w1193 = T22 4 items=["", "Zero Air", "Calib 1", "Calib 2", "Measure"] ("Requested Position")
                    n507 = local read "Mix_own_Calib_Gases"() -> (w1192:bool)
                    n508 = case shown="True" w1192 {
                      frame False {
                      }
                      frame True {
                        w1195 = 0.0 ("element")
                        n509 = Build Array("Clean_Air:Hi-Tec:Dem Volt", "GMU:Mains Divertor:Valve") -> (w1197:string[])
                        n510 = Build Array(w1195, w1195) -> (w1196:dbl[])
                        n511 = call "ASYNC_Adam_client.vi"("Values"=w1196, "Channel Names"=w1197) -> ()  [unwired: 1 in, 2 out]
                      }
                    }
                    n512 = call "Fast_FID_Valve_Control.vi"("Requested Position"=w1193) -> ()  [unwired: 7 out]
                  }
                }
              }
            }
          }
        }
      }
    }
    "Currently in Case" <- w18
  }
  "Error Messages" <- w12
